vi "Autonomous Independent.vi"   [LabVIEW 2017]
doc: "This VI is called when autonomous begins, and will automatically be terminated when autonomous ends. You can carry out timed or sensor driven robot movement independently without needing to return to the caller."
uses:
  <vilib>/Rock Robotics/WPI/Solenoid/WPI_SolenoidValue.ctl
  <vilib>/Rock Robotics/Network Tables/NT Read String.vi
  <vilib>/Rock Robotics/WPI/Solenoid/WPI_SolenoidSetEnum.vi
  Robot Global Data.vi
  <vilib>/Rock Robotics/WPI/Utilities/WPI_GetSetVariantRefNum.vi
  <vilib>/Rock Robotics/WPI/ThirdParty/Phoenix-LabVIEW/Motor Controller/Get/CTRE_Phoenix_MotorController_GetQuadratureData.vi
panel:
  # "Be sure to right-click and choose Data Operations>>Make Current Value default if you want to save the array values with the VI"
types:
  T1 = typedef "WPI_SolenoidValue.ctl" = enum16{"Off", "On", "Forward", "Reverse"}
  T2 = typedef "WPI_RobotDriveDevRef.ctl" = cluster{"DevStatus":errorcluster, "Motors[]":T3[], "Square Inputs":bool, "Max Output":dbl}
  T3 = typedef "WPI_MotorControlDeviceRef.ctl" = cluster{"DeviceStatus":errorcluster, "Type":T4, "PWM":cluster{"PWM Channel":T5, "DeadBand":T6}, "CAN":cluster{"Device Number":u8, "SetOutput VI Ref":variant, "GetOutput VI Ref":variant, "Enable VI Ref":variant, "Disable VI Ref":variant, "Data":variant}, "Invert":bool, "DIO PWM":cluster{"PWM \"Enable\" Channel":T5, "DIOChannel":T7, "PWM Rate":dbl}}
  T4 = typedef "WPI_MotorControlType.ctl" = enum16{"PWM", "CAN", "DIO PWM"}
  T5 = typedef "FPGA_DIOPWMChannel.ctl" = enum8{"PWM 0", "PWM 1", "PWM 2", "PWM 3", "PWM 4", "PWM 5", "PWM 6", "PWM 7", "PWM 8", "PWM 9", "PWM MXP 0", "PWM MXP 1", "PWM MXP 2", "PWM MXP 3", "PWM MXP 4", "PWM MXP 5", "PWM MXP 6", "PWM MXP 7", "PWM MXP 8", "PWM MXP 9", "Invalid"}
  T6 = typedef "WPI_PWMDeadband.ctl" = cluster{"Name":string, "maxPositivePwm":i32, "minPositivePwm":i32, "centerPwm":i32, "maxNegativePwm":i32, "minNegativePwm":i32, "angularRange":u16}
  T7 = typedef "FPGA_DIOChannel.ctl" = enum8{"DIO 0", "DIO 1", "DIO 2", "DIO 3", "DIO 4", "DIO 5", "DIO 6", "DIO 7", "DIO 8", "DIO 9", "DIO MXP 0", "DIO MXP 1", "DIO MXP 2", "DIO MXP 3", "DIO MXP 4", "DIO MXP 5", "DIO MXP 6", "DIO MXP 7", "DIO MXP 8", "DIO MXP 9", "DIO MXP 10", "DIO MXP 11", "DIO MXP 12", "DIO MXP 13", "DIO MXP 14", "DIO MXP 15", "SPI Port CS1", "SPI Port CS2", "SPI Port CS3", "SPI Port MISO", "SPI Port MOSI", "Invalid"}
  T8 = cluster{"Yaw":dbl, "Roll":dbl, "Pitch":dbl, "Heading":dbl, "Fused Heading":dbl}
  T9 = typedef "WPI_SolenoidDevRef.ctl" = cluster{"DevStatus":errorcluster, "Pneumatics Control Module":u8, "Forward Solenoid Channel":T10, "Reverse Solenoid Channel":T10}
  T10 = typedef "WPI_SolenoidChannel.ctl" = enum8{"Solenoid 0", "Solenoid 1", "Solenoid 2", "Solenoid 3", "Solenoid 4", "Solenoid 5", "Solenoid 6", "Solenoid 7", "Invalid"}
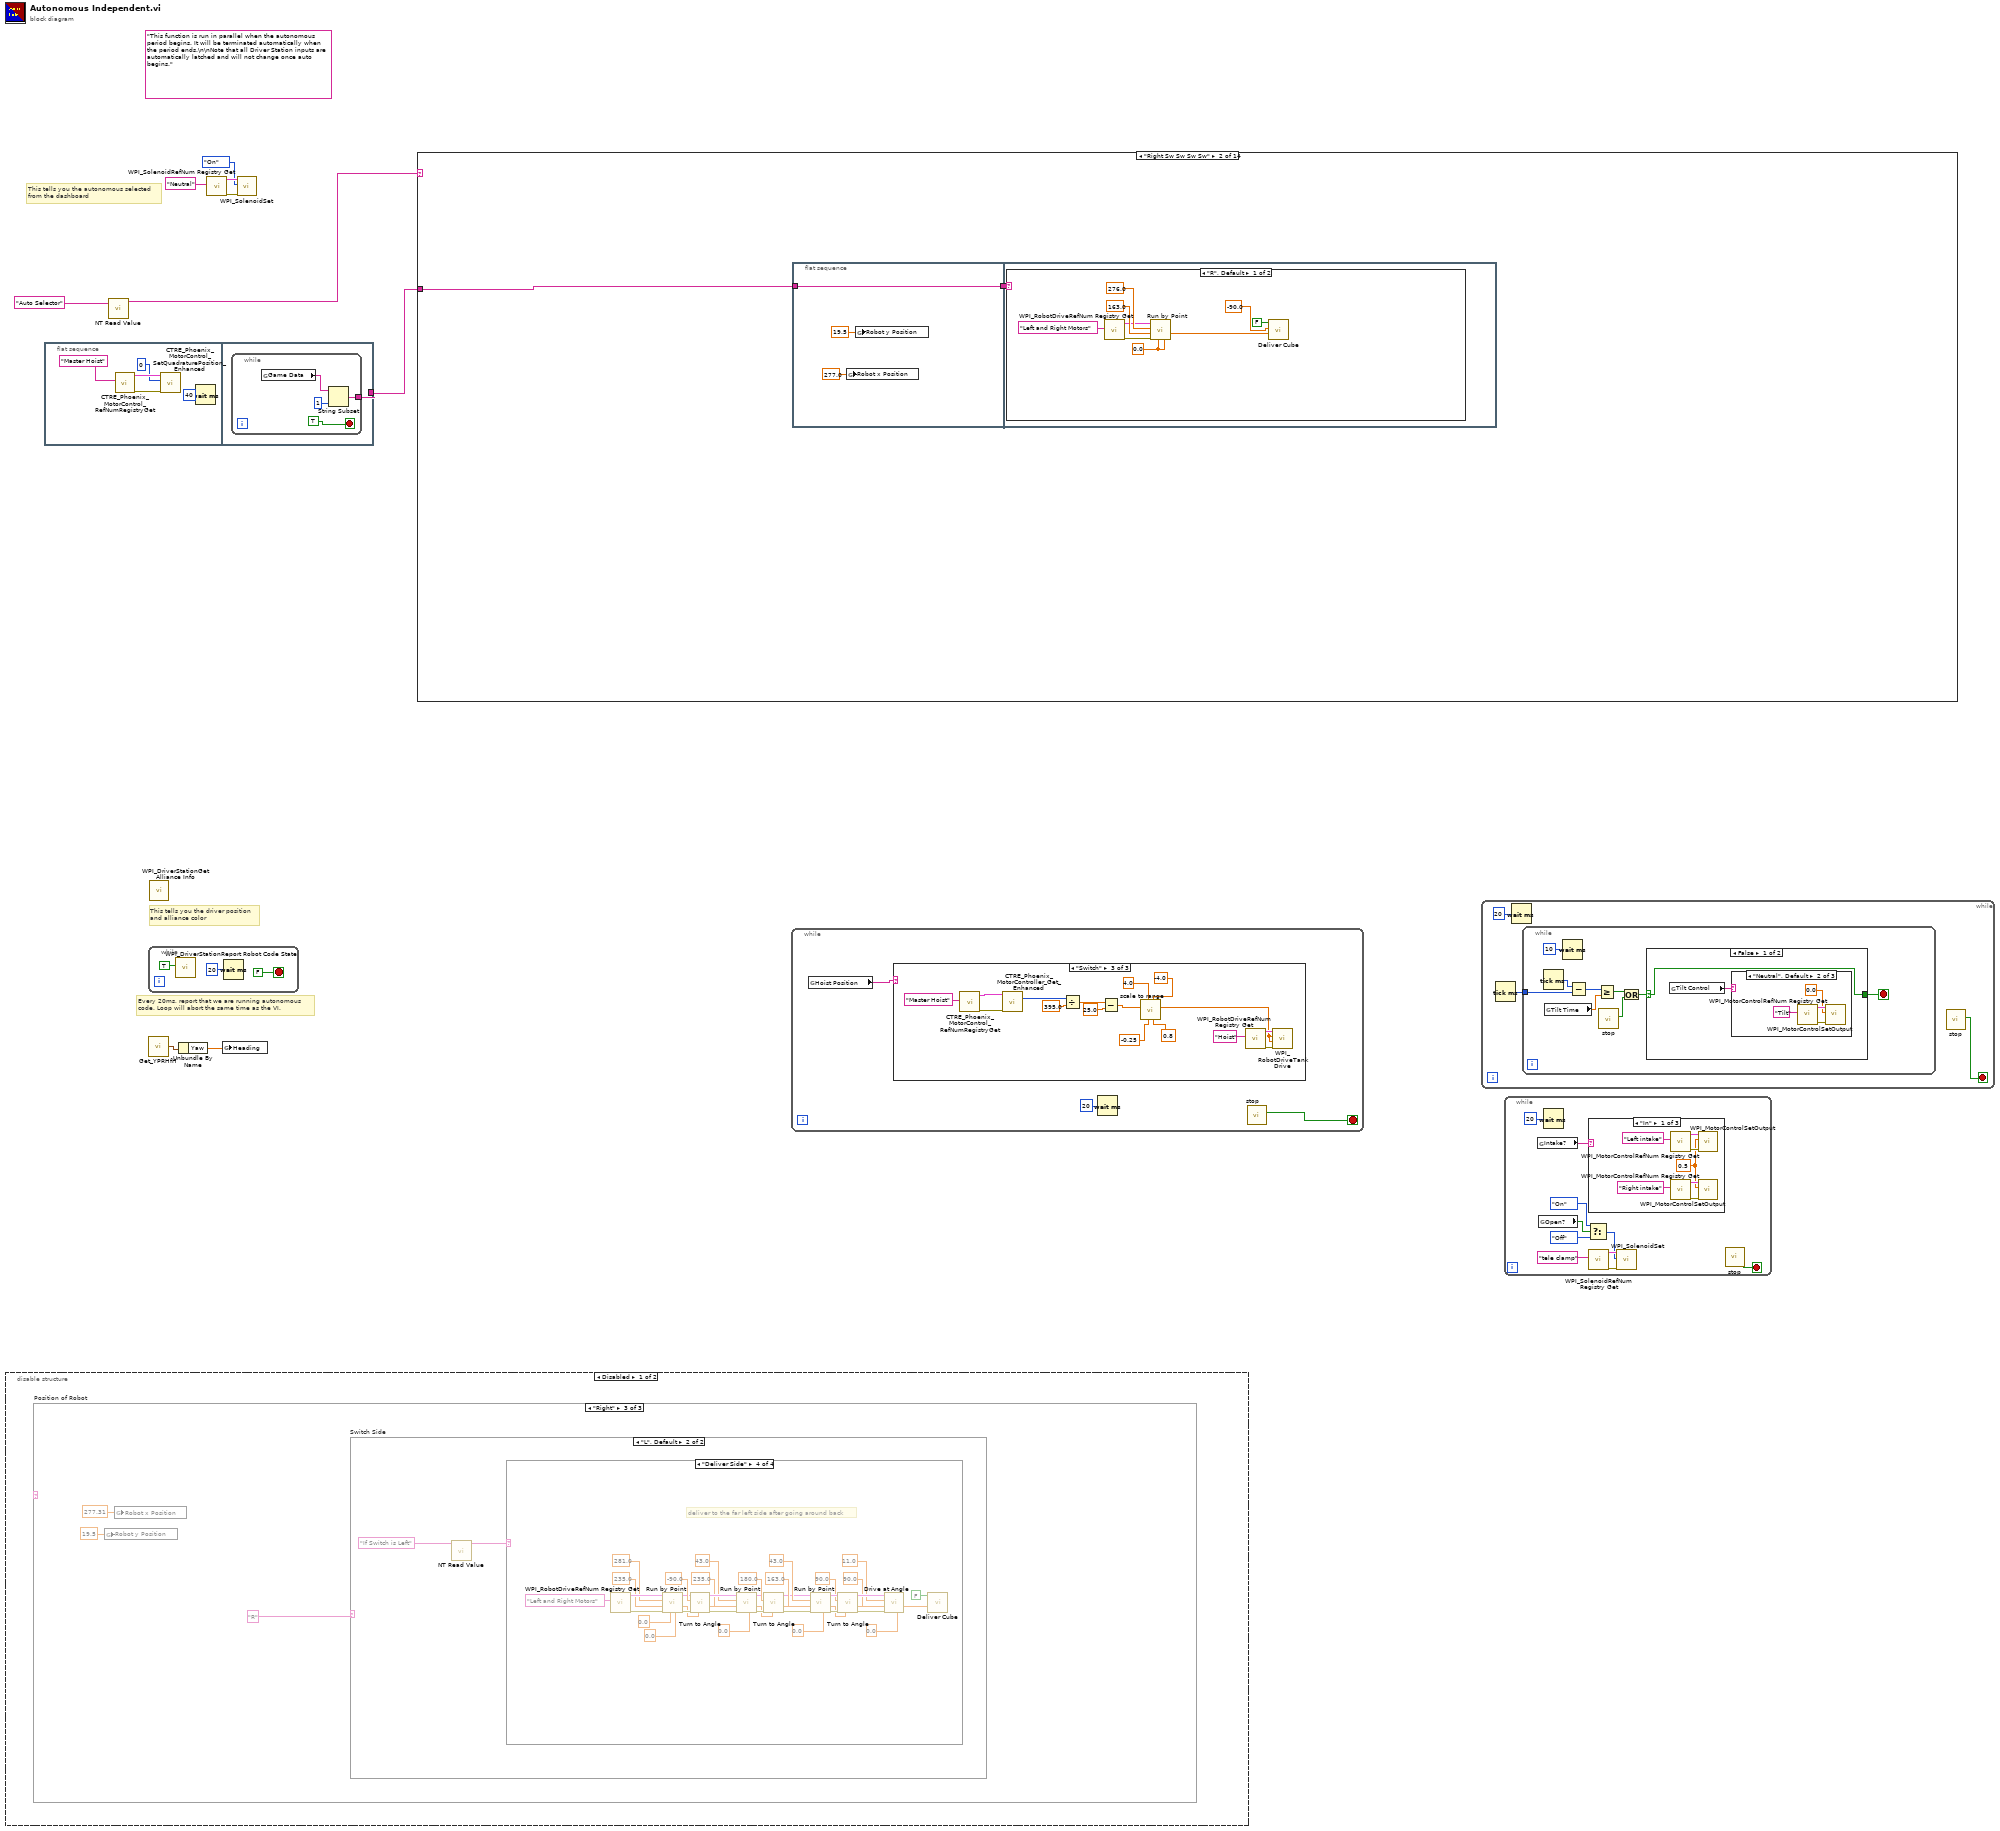
[diagram p0: block diagram]
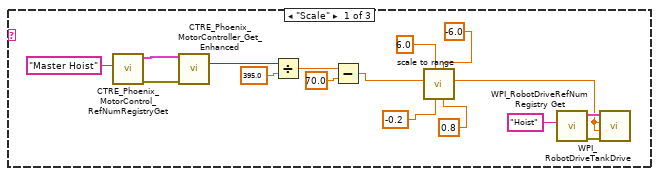
[diagram p2: hidden frame]
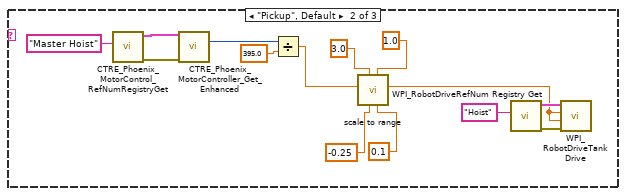
[diagram p3: hidden frame]
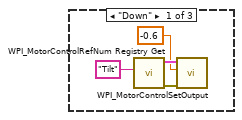
[diagram p4: hidden frame]
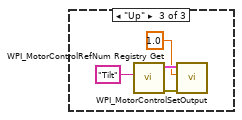
[diagram p5: hidden frame]
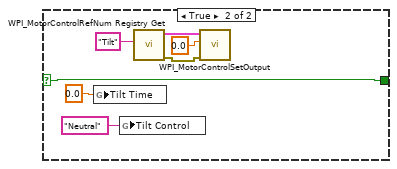
[diagram p6: hidden frame]
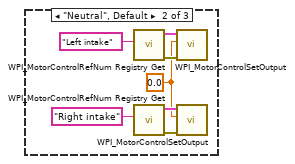
[diagram p7: hidden frame]
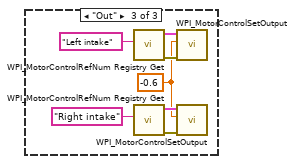
[diagram p8: hidden frame]
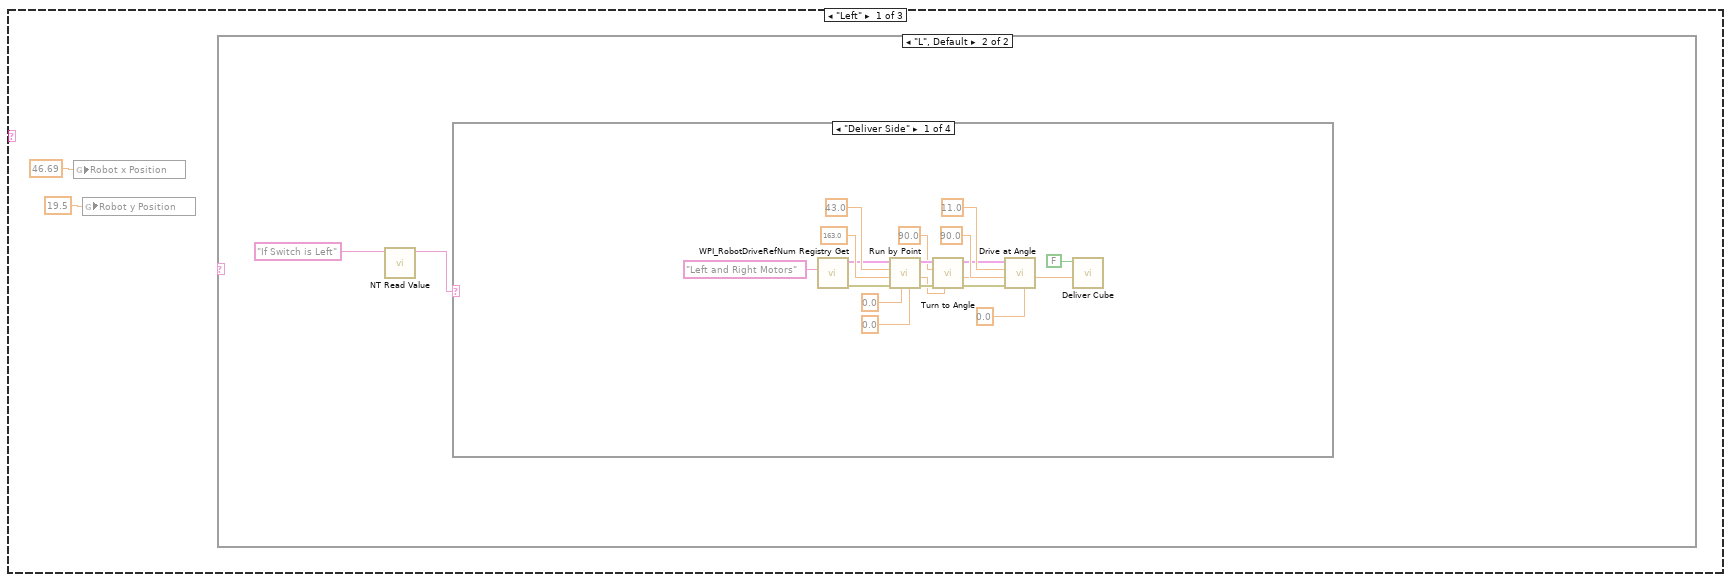
[diagram p9: hidden frame]
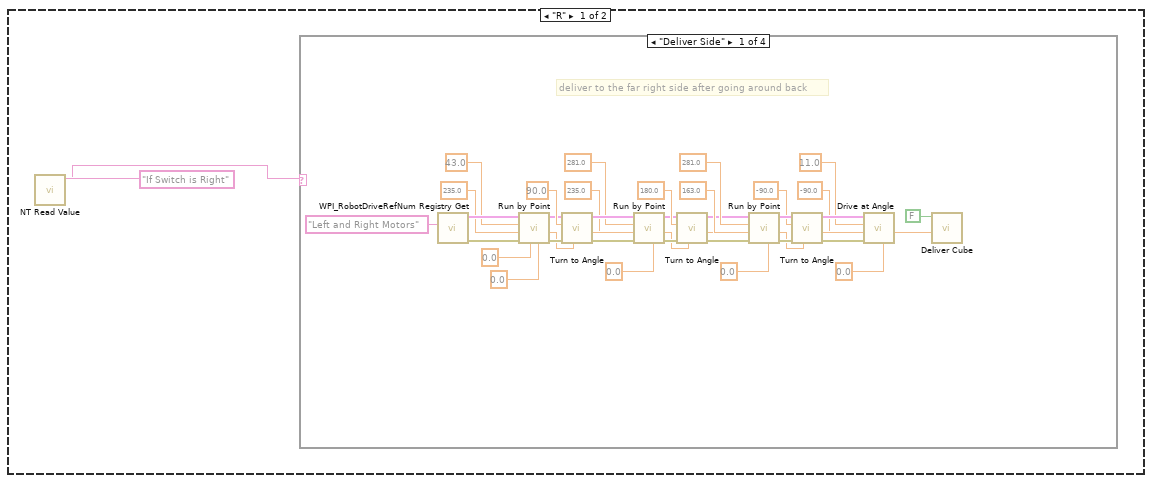
[diagram p10: hidden frame]
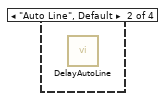
[diagram p11: hidden frame]
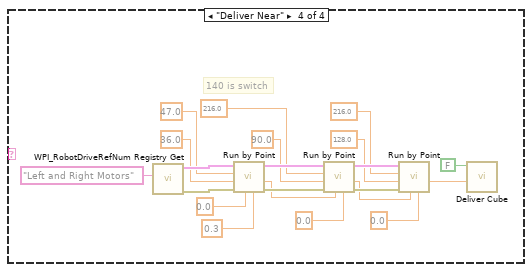
[diagram p13: hidden frame]
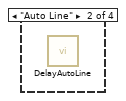
[diagram p14: hidden frame]
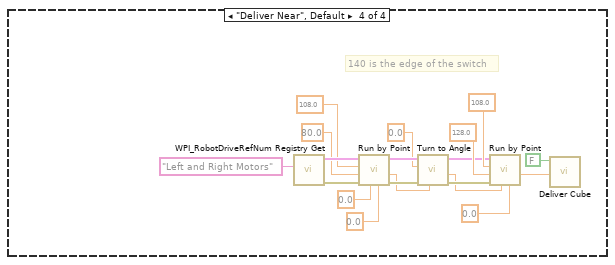
[diagram p16: hidden frame]
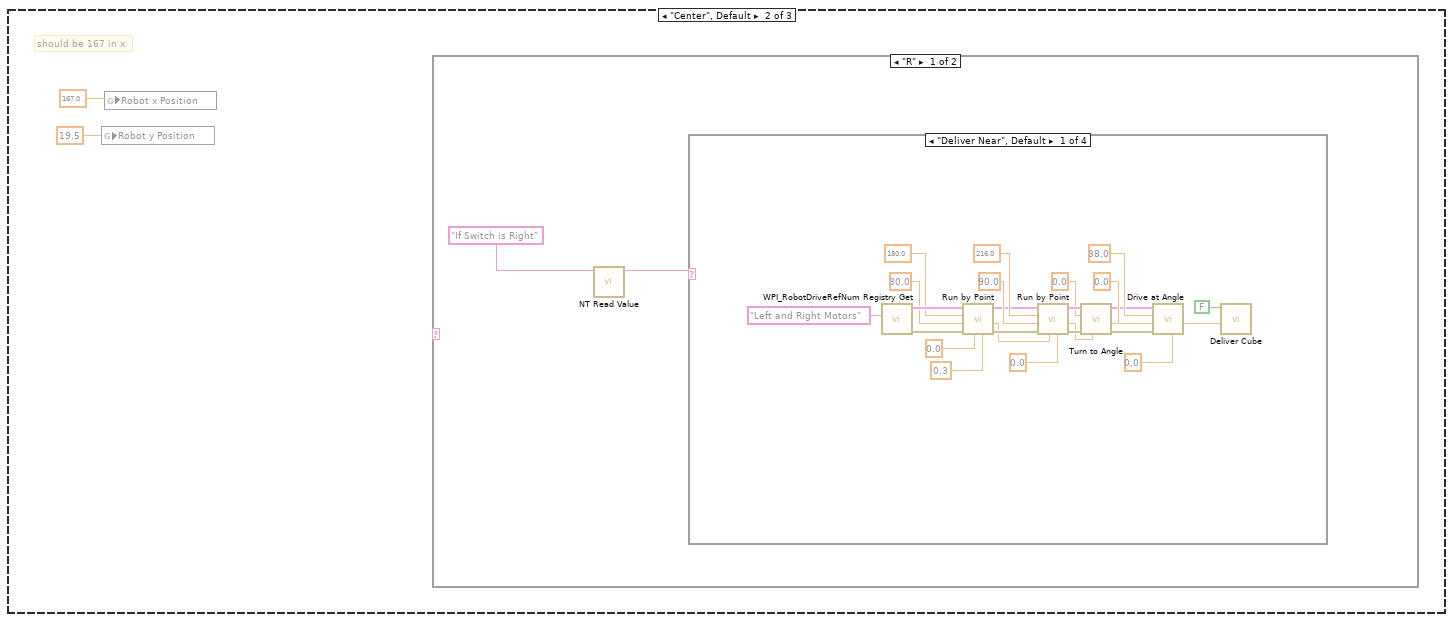
[diagram p17: hidden frame]
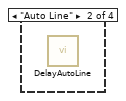
[diagram p18: hidden frame]
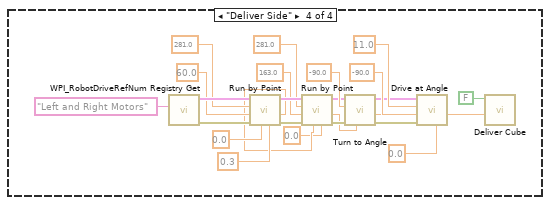
[diagram p20: hidden frame]
diagram:
  (unwired) "This function is run in parallel when the autonomous period begins. It will be terminated automatically when the period ends.\n\nNote that all Driver Station inputs are automatically latched and will not change once auto begins."
  # "This tells you the autonomous selected\nfrom the dashboard"
  # "Every 20ms, report that we are running autonomous\ncode. Loop will abort the same time as the VI."
  # "This tells you the driver position\nand alliance color"
  n1 = disable-structure shown="Disabled" {
    frame Disabled {
      n2 = case "Position of Robot" shown="\"Right\"" {
        selector: _ -> [_ _ _]
        frame "Left" {
          n3 = global write "Robot Global Data.vi" "Robot x Position"(46.69) -> ()
          n4 = global write "Robot Global Data.vi" "Robot y Position"(19.5) -> ()
          n5 = case shown="\"L\", Default" {
            selector: _ -> [_ _]
            frame "R" {
              n6 = call-poly <vilib>:"NT Read Value.vi"("Name"="If Switch is Right") -> ("String"=w12:string)  [unwired: 9 in, 1 out]
              n7 = case shown="\"Deliver Side\"" w12 {
                frame "Deliver Side" {
                  # "deliver to the far right side after going around back"
                  n8 = call <vilib>:"WPI_RobotDriveRefNum Registry Get.vi"("refnum name"="Left and Right Motors") -> ("error out"=w49:errorcluster, "RobotDriveDevRef"=w50:T2)  [unwired: 9 in]
                  n9 = call "Run by Point.vi"("end Power"=0.0 ("final power"), "Power in"=0.0 ("power in"), "error in (no error)"=w49, "y"=235.0, "x"=43.0, "RobotDriveDevRef"=w50) -> ("error out"=w40:errorcluster, "power out"=w39:dbl, "refnum"=w41:T2)  [unwired: 3 in]
                  n10 = call "Turn to Angle.vi"("in power"=w39, "error in (no error)"=w40, "Angle"=90.0 ("x"), "RobotDriveDevRef"=w41) -> ("error out"=w34:errorcluster, "out power"=w32:dbl, "ref Num"=w33:T2)  [unwired: 5 in]
                  n11 = call "Run by Point.vi"("end Power"=0.0, "Power in"=w32, "error in (no error)"=w34, "y"=235.0, "x"=281.0, "RobotDriveDevRef"=w33) -> ("error out"=w28:errorcluster, "power out"=w14:dbl, "refnum"=w29:T2)  [unwired: 3 in]
                  n12 = call "Turn to Angle.vi"("in power"=w14, "error in (no error)"=w28, "Angle"=180.0, "RobotDriveDevRef"=w29) -> ("error out"=w37:errorcluster, "out power"=w38:dbl, "ref Num"=w36:T2)  [unwired: 5 in]
                  n13 = call "Run by Point.vi"("end Power"=0.0 ("final power"), "Power in"=w38, "error in (no error)"=w37, "y"=163.0, "x"=281.0, "RobotDriveDevRef"=w36) -> ("error out"=w25:errorcluster, "power out"=w24:dbl, "refnum"=w26:T2)  [unwired: 3 in]
                  n14 = call "Turn to Angle.vi"("in power"=w24, "error in (no error)"=w25, "Angle"=-90.0, "RobotDriveDevRef"=w26) -> ("error out"=w21:errorcluster, "out power"=w20:dbl, "ref Num"=w22:T2)  [unwired: 5 in]
                  n15 = call "Drive at Angle.vi"("end power"=0.0, "Begin power"=w20, "error in (no error)"=w21, "Angle"=-90.0, "Distance"=11.0, "RobotDriveDevRef"=w22) -> ("power out"=w16:dbl)  [unwired: 3 in, 2 out]
                  n16 = call "Deliver Cube.vi"("run?"=w16, "Scale?"=FALSE) -> ()  [unwired: 9 in, 1 out]
                }
                frame "Auto Line", Default {
                  n17 = call "DelayAutoLine.vi"() -> ()  [unwired: 12 in]
                }
                frame "Scale" {
                }
                frame "Deliver Near" {
                  # "140 is switch"
                  n18 = call <vilib>:"WPI_RobotDriveRefNum Registry Get.vi"("refnum name"="Left and Right Motors") -> ("error out"=w70:errorcluster, "RobotDriveDevRef"=w71:T2)  [unwired: 9 in]
                  n19 = call "Run by Point.vi"("end Power"=0.3 ("final power"), "Power in"=0.0 ("power in"), "error in (no error)"=w70, "y"=36.0, "x"=47.0, "RobotDriveDevRef"=w71) -> ("error out"=w66:errorcluster, "power out"=w57:dbl, "refnum"=w67:T2)  [unwired: 3 in]
                  n20 = call "Run by Point.vi"("end Power"=0.0 ("final power"), "Power in"=w57, "error in (no error)"=w66, "y"=90.0, "x"=216.0, "RobotDriveDevRef"=w67) -> ("error out"=w64:errorcluster, "power out"=w63:dbl, "refnum"=w65:T2)  [unwired: 3 in]
                  n21 = call "Run by Point.vi"("end Power"=0.0 ("final power"), "Power in"=w63, "error in (no error)"=w64, "y"=128.0, "x"=216.0, "RobotDriveDevRef"=w65) -> ("power out"=w55:dbl)  [unwired: 3 in, 2 out]
                  n22 = call "Deliver Cube.vi"("run?"=w55, "Scale?"=FALSE) -> ()  [unwired: 9 in, 1 out]
                }
              }
            }
            frame "L", Default {
              n23 = call-poly <vilib>:"NT Read Value.vi"("Name"="If Switch is Left") -> ("String"=w74:string)  [unwired: 9 in, 1 out]
              n24 = case shown="\"Deliver Side\"" w74 {
                frame "Deliver Side" {
                  n25 = call <vilib>:"WPI_RobotDriveRefNum Registry Get.vi"("refnum name"="Left and Right Motors") -> ("error out"=w77:errorcluster, "RobotDriveDevRef"=w78:T2)  [unwired: 9 in]
                  n26 = call "Run by Point.vi"("end Power"=0.0 ("final power"), "Power in"=0.0, "error in (no error)"=w77, "y"=163.0 ("x"), "x"=43.0 ("y"), "RobotDriveDevRef"=w78) -> ("error out"=w87:errorcluster, "power out"=w82:dbl, "refnum"=w84:T2)  [unwired: 3 in]
                  n27 = call "Turn to Angle.vi"("in power"=w82, "error in (no error)"=w87, "Angle"=90.0, "RobotDriveDevRef"=w84) -> ("error out"=w86:errorcluster, "out power"=w81:dbl, "ref Num"=w85:T2)  [unwired: 5 in]
                  n28 = call "Drive at Angle.vi"("end power"=0.0, "Begin power"=w81, "error in (no error)"=w86, "Angle"=90.0, "Distance"=11.0, "RobotDriveDevRef"=w85) -> ("power out"=w80:dbl)  [unwired: 3 in, 2 out]
                  n29 = call "Deliver Cube.vi"("run?"=w80, "Scale?"=FALSE) -> ()  [unwired: 9 in, 1 out]
                }
                frame "Auto Line" {
                  n30 = call "DelayAutoLine.vi"() -> ()  [unwired: 12 in]
                }
                frame "Scale" {
                }
                frame "Deliver Near", Default {
                  # "140 is the edge of the switch"
                  n31 = call <vilib>:"WPI_RobotDriveRefNum Registry Get.vi"("refnum name"="Left and Right Motors") -> ("error out"=w108:errorcluster, "RobotDriveDevRef"=w109:T2)  [unwired: 9 in]
                  n32 = call "Run by Point.vi"("end Power"=0.0 ("end power"), "Power in"=0.0 ("end speed"), "error in (no error)"=w108, "y"=80.0 ("Angle"), "x"=108.0 ("Distance"), "RobotDriveDevRef"=w109) -> ("error out"=w100:errorcluster, "power out"=w99:dbl, "refnum"=w103:T2)  [unwired: 3 in]
                  n33 = call "Turn to Angle.vi"("in power"=w99, "error in (no error)"=w100, "Angle"=0.0 ("y"), "RobotDriveDevRef"=w103) -> ("error out"=w101:errorcluster, "out power"=w97:dbl, "ref Num"=w102:T2)  [unwired: 5 in]
                  n34 = call "Run by Point.vi"("end Power"=0.0, "Power in"=w97, "error in (no error)"=w101, "y"=128.0, "x"=108.0, "RobotDriveDevRef"=w102) -> ("power out"=w96:dbl)  [unwired: 3 in, 2 out]
                  n35 = call "Deliver Cube.vi"("run?"=w96, "Scale?"=FALSE) -> ()  [unwired: 9 in, 1 out]
                }
              }
            }
          }
        }
        frame "Center", Default {
          # "should be 167 in x"
          n36 = global write "Robot Global Data.vi" "Robot y Position"(19.5) -> ()
          n37 = global write "Robot Global Data.vi" "Robot x Position"(167.0) -> ()
          n38 = case shown="\"R\"" {
            selector: _ -> [_ _]
            frame "R" {
              n39 = call-poly <vilib>:"NT Read Value.vi"("Name"="If Switch is Right") -> ("String"=w116:string)  [unwired: 9 in, 1 out]
              n40 = case shown="\"Deliver Near\", Default" w116 {
                frame "Deliver Near", Default {
                  n41 = call <vilib>:"WPI_RobotDriveRefNum Registry Get.vi"("refnum name"="Left and Right Motors") -> ("error out"=w133:errorcluster, "RobotDriveDevRef"=w134:T2)  [unwired: 9 in]
                  n42 = call "Run by Point.vi"("end Power"=0.3 ("Power in"), "Power in"=0.0, "error in (no error)"=w133, "y"=30.0, "x"=180.0, "RobotDriveDevRef"=w134) -> ("error out"=w132:errorcluster, "power out"=w130:dbl, "refnum"=w131:T2)  [unwired: 3 in]
                  n43 = call "Run by Point.vi"("end Power"=0.0, "Power in"=w130, "error in (no error)"=w132, "y"=90.0, "x"=216.0, "RobotDriveDevRef"=w131) -> ("error out"=w125:errorcluster, "power out"=w123:dbl, "refnum"=w124:T2)  [unwired: 3 in]
                  n44 = call "Turn to Angle.vi"("in power"=w123, "error in (no error)"=w125, "Angle"=0.0, "RobotDriveDevRef"=w124) -> ("error out"=w121:errorcluster, "out power"=w119:dbl, "ref Num"=w120:T2)  [unwired: 5 in]
                  n45 = call "Drive at Angle.vi"("end power"=0.0 ("final power"), "Begin power"=w119, "error in (no error)"=w121, "Angle"=0.0 ("x"), "Distance"=38.0 ("y"), "RobotDriveDevRef"=w120) -> ("power out"=w118:dbl)  [unwired: 3 in, 2 out]
                  n46 = call "Deliver Cube.vi"("run?"=w118, "Scale?"=FALSE) -> ()  [unwired: 9 in, 1 out]
                }
                frame "Auto Line" {
                  n47 = call "DelayAutoLine.vi"() -> ()  [unwired: 12 in]
                }
                frame "Scale" {
                }
                frame "Deliver Side" {
                  n48 = call <vilib>:"WPI_RobotDriveRefNum Registry Get.vi"("refnum name"="Left and Right Motors") -> ("error out"=w156:errorcluster, "RobotDriveDevRef"=w166:T2)  [unwired: 9 in]
                  n49 = call "Run by Point.vi"("end Power"=0.3 ("final power"), "Power in"=0.0 ("power in"), "error in (no error)"=w156, "y"=60.0, "x"=281.0, "RobotDriveDevRef"=w166) -> ("error out"=w151:errorcluster, "power out"=w150:dbl, "refnum"=w152:T2)  [unwired: 3 in]
                  n50 = call "Run by Point.vi"("end Power"=0.0, "Power in"=w150, "error in (no error)"=w151, "y"=163.0, "x"=281.0, "RobotDriveDevRef"=w152) -> ("error out"=w146:errorcluster, "power out"=w145:dbl, "refnum"=w147:T2)  [unwired: 3 in]
                  n51 = call "Turn to Angle.vi"("in power"=w145, "error in (no error)"=w146, "Angle"=-90.0 ("x"), "RobotDriveDevRef"=w147) -> ("error out"=w153:errorcluster, "out power"=w144:dbl, "ref Num"=w154:T2)  [unwired: 5 in]
                  n52 = call "Drive at Angle.vi"("end power"=0.0, "Begin power"=w144, "error in (no error)"=w153, "Angle"=-90.0, "Distance"=11.0, "RobotDriveDevRef"=w154) -> ("power out"=w158:dbl)  [unwired: 3 in, 2 out]
                  n53 = call "Deliver Cube.vi"("run?"=w158, "Scale?"=FALSE) -> ()  [unwired: 9 in, 1 out]
                }
              }
            }
            frame "L", Default {
              n54 = call-poly <vilib>:"NT Read Value.vi"("Name"="If Switch is Left") -> ("String"=w168:string)  [unwired: 9 in, 1 out]
              n55 = case shown="\"Deliver Near\", Default" w168 {
                frame "Deliver Near", Default {
                  n56 = call <vilib>:"WPI_RobotDriveRefNum Registry Get.vi"("refnum name"="Left and Right Motors") -> ("error out"=w185:errorcluster, "RobotDriveDevRef"=w186:T2)  [unwired: 9 in]
                  n57 = call "Run by Point.vi"("end Power"=0.3 ("Power in"), "Power in"=0.0, "error in (no error)"=w185, "y"=30.0, "x"=150.0, "RobotDriveDevRef"=w186) -> ("error out"=w184:errorcluster, "power out"=w182:dbl, "refnum"=w183:T2)  [unwired: 3 in]
                  n58 = call "Run by Point.vi"("end Power"=0.0, "Power in"=w182, "error in (no error)"=w184, "y"=90.0, "x"=108.0, "RobotDriveDevRef"=w183) -> ("error out"=w177:errorcluster, "power out"=w175:dbl, "refnum"=w176:T2)  [unwired: 3 in]
                  n59 = call "Turn to Angle.vi"("in power"=w175, "error in (no error)"=w177, "Angle"=0.0, "RobotDriveDevRef"=w176) -> ("error out"=w173:errorcluster, "out power"=w171:dbl, "ref Num"=w172:T2)  [unwired: 5 in]
                  n60 = call "Drive at Angle.vi"("end power"=0.0 ("final power"), "Begin power"=w171, "error in (no error)"=w173, "Angle"=0.0 ("x"), "Distance"=38.0 ("y"), "RobotDriveDevRef"=w172) -> ("power out"=w170:dbl)  [unwired: 3 in, 2 out]
                  n61 = call "Deliver Cube.vi"("run?"=w170, "Scale?"=FALSE) -> ()  [unwired: 9 in, 1 out]
                }
                frame "Auto Line" {
                  n62 = call "DelayAutoLine.vi"() -> ()  [unwired: 12 in]
                }
                frame "Scale" {
                }
                frame "Deliver Side" {
                  n63 = call <vilib>:"WPI_RobotDriveRefNum Registry Get.vi"("refnum name"="Left and Right Motors") -> ("error out"=w208:errorcluster, "RobotDriveDevRef"=w218:T2)  [unwired: 9 in]
                  n64 = call "Run by Point.vi"("end Power"=0.3 ("final power"), "Power in"=0.0 ("power in"), "error in (no error)"=w208, "y"=60.0, "x"=43.0, "RobotDriveDevRef"=w218) -> ("error out"=w203:errorcluster, "power out"=w202:dbl, "refnum"=w204:T2)  [unwired: 3 in]
                  n65 = call "Run by Point.vi"("end Power"=0.0, "Power in"=w202, "error in (no error)"=w203, "y"=163.0, "x"=43.0, "RobotDriveDevRef"=w204) -> ("error out"=w198:errorcluster, "power out"=w197:dbl, "refnum"=w199:T2)  [unwired: 3 in]
                  n66 = call "Turn to Angle.vi"("in power"=w197, "error in (no error)"=w198, "Angle"=90.0 ("x"), "RobotDriveDevRef"=w199) -> ("error out"=w205:errorcluster, "out power"=w196:dbl, "ref Num"=w206:T2)  [unwired: 5 in]
                  n67 = call "Drive at Angle.vi"("end power"=0.0, "Begin power"=w196, "error in (no error)"=w205, "Angle"=90.0, "Distance"=11.0, "RobotDriveDevRef"=w206) -> ("power out"=w210:dbl)  [unwired: 3 in, 2 out]
                  n68 = call "Deliver Cube.vi"("run?"=w210, "Scale?"=FALSE) -> ()  [unwired: 9 in, 1 out]
                }
              }
            }
          }
        }
        frame "Right" {
          n69 = global write "Robot Global Data.vi" "Robot y Position"(19.5) -> ()
          n70 = global write "Robot Global Data.vi" "Robot x Position"(277.31) -> ()
          n71 = case "Switch Side" shown="\"L\", Default" "R" {
            frame "R" {
              n72 = call-poly <vilib>:"NT Read Value.vi"("Name"="If Switch is Right") -> ()  [unwired: 9 in, 2 out]
              n73 = case "What Program to Run" shown="\"Deliver Side\"" "Auto Line" {
                frame "Deliver Near", Default {
                  n74 = call <vilib>:"WPI_RobotDriveRefNum Registry Get.vi"("refnum name"="Left and Right Motors") -> ("error out"=w240:errorcluster, "RobotDriveDevRef"=w241:T2)  [unwired: 9 in]
                  n75 = call "Run by Point.vi"("end Power"=0.3 ("Power in"), "Power in"=0.0, "error in (no error)"=w240, "y"=30.0, "x"=250.0, "RobotDriveDevRef"=w241) -> ("error out"=w239:errorcluster, "power out"=w237:dbl, "refnum"=w238:T2)  [unwired: 3 in]
                  n76 = call "Run by Point.vi"("end Power"=0.0, "Power in"=w237, "error in (no error)"=w239, "y"=90.0, "x"=216.0, "RobotDriveDevRef"=w238) -> ("error out"=w232:errorcluster, "power out"=w230:dbl, "refnum"=w231:T2)  [unwired: 3 in]
                  n77 = call "Turn to Angle.vi"("in power"=w230, "error in (no error)"=w232, "Angle"=0.0, "RobotDriveDevRef"=w231) -> ("error out"=w228:errorcluster, "out power"=w226:dbl, "ref Num"=w227:T2)  [unwired: 5 in]
                  n78 = call "Drive at Angle.vi"("end power"=0.0 ("final power"), "Begin power"=w226, "error in (no error)"=w228, "Angle"=0.0 ("x"), "Distance"=38.0 ("y"), "RobotDriveDevRef"=w227) -> ("power out"=w225:dbl)  [unwired: 3 in, 2 out]
                  n79 = call "Deliver Cube.vi"("run?"=w225, "Scale?"=FALSE) -> ()  [unwired: 9 in, 1 out]
                }
                frame "Auto Line" {
                  n80 = call "DelayAutoLine.vi"() -> ()  [unwired: 12 in]
                }
                frame "Scale" {
                }
                frame "Deliver Side" {
                  n81 = call <vilib>:"WPI_RobotDriveRefNum Registry Get.vi"("refnum name"="Left and Right Motors") -> ("error out"=w250:errorcluster, "RobotDriveDevRef"=w251:T2)  [unwired: 9 in]
                  n82 = call "Run by Point.vi"("end Power"=0.0, "error in (no error)"=w250, "y"=163.0, "x"=281.0, "RobotDriveDevRef"=w251) -> ("error out"=w255:errorcluster, "power out"=w254:dbl, "refnum"=w256:T2)  [unwired: 4 in]
                  n83 = call "Turn to Angle.vi"("in power"=w254, "error in (no error)"=w255, "Angle"=-90.0 ("x"), "RobotDriveDevRef"=w256) -> ("error out"=w259:errorcluster, "out power"=w253:dbl, "ref Num"=w260:T2)  [unwired: 5 in]
                  n84 = call "Drive at Angle.vi"("end power"=0.0, "Begin power"=w253, "error in (no error)"=w259, "Angle"=-90.0, "Distance"=11.0, "RobotDriveDevRef"=w260) -> ("power out"=w263:dbl)  [unwired: 3 in, 2 out]
                  n85 = call "Deliver Cube.vi"("run?"=w263, "Scale?"=FALSE) -> ()  [unwired: 9 in, 1 out]
                }
              }
            }
            frame "L", Default {
              n86 = call-poly <vilib>:"NT Read Value.vi"("Name"="If Switch is Left") -> ("String"=w268:string)  [unwired: 9 in, 1 out]
              n87 = case shown="\"Deliver Side\"" w268 {
                frame "Deliver Near" {
                  # "140 is switch"
                  n88 = call <vilib>:"WPI_RobotDriveRefNum Registry Get.vi"("refnum name"="Left and Right Motors") -> ("error out"=w287:errorcluster, "RobotDriveDevRef"=w288:T2)  [unwired: 9 in]
                  n89 = call "Run by Point.vi"("end Power"=0.3 ("final power"), "Power in"=0.0 ("power in"), "error in (no error)"=w287, "y"=45.0, "x"=108.0, "RobotDriveDevRef"=w288) -> ("error out"=w283:errorcluster, "power out"=w274:dbl, "refnum"=w284:T2)  [unwired: 3 in]
                  n90 = call "Run by Point.vi"("end Power"=0.3 ("final power"), "Power in"=w274, "error in (no error)"=w283, "y"=90.0, "x"=108.0, "RobotDriveDevRef"=w284) -> ("error out"=w281:errorcluster, "power out"=w280:dbl, "refnum"=w282:T2)  [unwired: 3 in]
                  n91 = call "Drive at Angle.vi"("end power"=0.0 ("final power"), "Begin power"=w280, "error in (no error)"=w281, "Angle"=0.0 ("y"), "Distance"=38.0 ("x"), "RobotDriveDevRef"=w282) -> ("power out"=w272:dbl)  [unwired: 3 in, 2 out]
                  n92 = call "Deliver Cube.vi"("run?"=w272, "Scale?"=FALSE) -> ()  [unwired: 9 in, 1 out]
                }
                frame "Auto Line", Default {
                  n93 = call "DelayAutoLine.vi"() -> ()  [unwired: 12 in]
                }
                frame "Scale" {
                }
                frame "Deliver Side" {
                  # "deliver to the far left side after going around back"
                  n94 = call <vilib>:"WPI_RobotDriveRefNum Registry Get.vi"("refnum name"="Left and Right Motors") -> ("error out"=w326:errorcluster, "RobotDriveDevRef"=w327:T2)  [unwired: 9 in]
                  n95 = call "Run by Point.vi"("end Power"=0.0 ("final power"), "Power in"=0.0 ("power in"), "error in (no error)"=w326, "y"=235.0, "x"=281.0, "RobotDriveDevRef"=w327) -> ("error out"=w317:errorcluster, "power out"=w316:dbl, "refnum"=w318:T2)  [unwired: 3 in]
                  n96 = call "Turn to Angle.vi"("in power"=w316, "error in (no error)"=w317, "Angle"=-90.0 ("x"), "RobotDriveDevRef"=w318) -> ("error out"=w311:errorcluster, "out power"=w309:dbl, "ref Num"=w310:T2)  [unwired: 5 in]
                  n97 = call "Run by Point.vi"("end Power"=0.0, "Power in"=w309, "error in (no error)"=w311, "y"=235.0, "x"=43.0, "RobotDriveDevRef"=w310) -> ("error out"=w305:errorcluster, "power out"=w291:dbl, "refnum"=w306:T2)  [unwired: 3 in]
                  n98 = call "Turn to Angle.vi"("in power"=w291, "error in (no error)"=w305, "Angle"=180.0, "RobotDriveDevRef"=w306) -> ("error out"=w314:errorcluster, "out power"=w315:dbl, "ref Num"=w313:T2)  [unwired: 5 in]
                  n99 = call "Run by Point.vi"("end Power"=0.0 ("final power"), "Power in"=w315, "error in (no error)"=w314, "y"=163.0, "x"=43.0, "RobotDriveDevRef"=w313) -> ("error out"=w302:errorcluster, "power out"=w301:dbl, "refnum"=w303:T2)  [unwired: 3 in]
                  n100 = call "Turn to Angle.vi"("in power"=w301, "error in (no error)"=w302, "Angle"=90.0, "RobotDriveDevRef"=w303) -> ("error out"=w298:errorcluster, "out power"=w297:dbl, "ref Num"=w299:T2)  [unwired: 5 in]
                  n101 = call "Drive at Angle.vi"("end power"=0.0, "Begin power"=w297, "error in (no error)"=w298, "Angle"=90.0, "Distance"=11.0, "RobotDriveDevRef"=w299) -> ("power out"=w293:dbl)  [unwired: 3 in, 2 out]
                  n102 = call "Deliver Cube.vi"("run?"=w293, "Scale?"=FALSE) -> ()  [unwired: 9 in, 1 out]
                }
              }
            }
          }
        }
      }
    }
    frame Enabled {
    }
  }
  n103 = flat-sequence {
    tunnel: [w335] -> w1
    frame #0 {
      n104 = call <vilib>:"CTRE_Phoenix_MotorControl_RefNumRegistryGet.vi"("refnum name"="Master Hoist") -> ("error out"=w333:errorcluster, "PhoenixMotorControlDevRef"=w332:T3)  [unwired: 9 in]
      n105 = call <vilib>:"CTRE_Phoenix_MotorControl_SetQuadraturePosition_Enhanced.vi"("error in (no error)"=w333, "New Position"=0, "PhoenixMotorControlDevRef"=w332) -> ()  [unwired: 7 in, 2 out]
      n106 = Wait (ms)(milliseconds to wait=u32 40) -> ()  [unwired: 1 out]
    }
    frame #1 {
      n107 = while {
        tunnel: [w338] -> w335
        stop <- TRUE stop-if-true
        n108 = global read "Robot Global Data.vi" "Game Data"() -> (w337:string)
        n109 = String Subset(string=w337, length (rest)=1 ("length (rest)")) -> (substring=w338:string)  [unwired: 1 in]
      }
    }
  }
  n110 = call-poly <vilib>:"NT Read Value.vi"("Name"="Auto Selector") -> ("String"=w2:string)  [unwired: 9 in, 1 out]
  n111 = while {
    stop <- FALSE stop-if-true
    n112 = call <vilib>:"WPI_DriverStationReport Robot Code State.vi"("Autonomous"=TRUE) -> ()  [unwired: 10 in, 1 out]
    n113 = Wait (ms)(milliseconds to wait=u32 20) -> ()  [unwired: 1 out]
  }
  n114 = call <vilib>:"Get_YPRHfH.vi"() -> ("YRPHfH"=w7:T8)  [unwired: 11 in]
  n115 = call <vilib>:"WPI_DriverStationGet Alliance Info.vi"() -> ()  [unwired: 12 out]
  n116 = Unbundle By Name(w7) -> ("Yaw"=w8:dbl)
  n117 = call <vilib>:"WPI_SolenoidRefNum Registry Get.vi"("refnum name"="Neutral") -> ("error out"=w6:errorcluster, "SolenoidDevRef"=w5:T9)  [unwired: 9 in]
  n118 = global write "Robot Global Data.vi" "Heading"(w8) -> ()
  n119 = call-poly <vilib>:"WPI_SolenoidSet.vi"("error in (no error)"=w6, "Value"=WPI_SolenoidValue."On", "SolenoidDevRef"=w5) -> ()  [unwired: 7 in, 2 out]
  n120 = case shown="\"Right Sw Sw Sw Sw\"" w2 {
    tunnel: w1 -> [w344 w370 _ w417 w432 w446 w451 _ _ w579 w644 w707 w770 w833]
    frame "Center" {
      n121 = flat-sequence {
        tunnel: w344 -> [w347]
        tunnel: [w347] -> w343
        tunnel: w343 -> [w348]
        frame #0 {
          n122 = global write "Robot Global Data.vi" "Robot y Position"(19.5) -> ()
          n123 = global write "Robot Global Data.vi" "Robot x Position"(167.0) -> ()
        }
        frame #1 {
          n124 = case shown="\"L\", Default" w348 {
            frame "R" {
              n125 = call <vilib>:"WPI_RobotDriveRefNum Registry Get.vi"("refnum name"="Left and Right Motors") -> ("error out"=w354:errorcluster, "RobotDriveDevRef"=w355:T2)  [unwired: 9 in]
              n126 = call "Run by Point.vi"("end Power"=0.0, "Power in"=0.0, "error in (no error)"=w354, "y"=103.0, "x"=216.0, "RobotDriveDevRef"=w355) -> ("power out"=w353:dbl)  [unwired: 3 in, 2 out]
              n127 = call "Deliver Cube.vi"("run?"=w353, "Angle"=0.0, "Scale?"=FALSE) -> ()  [unwired: 8 in, 1 out]
            }
            frame "L", Default {
              n128 = call <vilib>:"WPI_RobotDriveRefNum Registry Get.vi"("refnum name"="Left and Right Motors") -> ("error out"=w364:errorcluster, "RobotDriveDevRef"=w365:T2)  [unwired: 9 in]
              n129 = call "Run by Point.vi"("end Power"=0.0, "Power in"=0.0, "error in (no error)"=w364, "y"=103.0, "x"=108.0, "RobotDriveDevRef"=w365) -> ("power out"=w359:dbl)  [unwired: 3 in, 2 out]
              n130 = call "Deliver Cube.vi"("run?"=w359, "Angle"=0.0, "Scale?"=FALSE) -> ()  [unwired: 8 in, 1 out]
            }
          }
        }
      }
    }
    frame "Right Sw Sw Sw Sw" {
      n131 = flat-sequence {
        tunnel: w370 -> [w373]
        tunnel: [w373] -> w369
        tunnel: w369 -> [w374]
        frame #0 {
          n132 = global write "Robot Global Data.vi" "Robot x Position"(277.0) -> ()
          n133 = global write "Robot Global Data.vi" "Robot y Position"(19.5) -> ()
        }
        frame #1 {
          n134 = case shown="\"R\", Default" w374 {
            frame "R", Default {
              w376 = 0.0 ("end Power")
              n135 = call <vilib>:"WPI_RobotDriveRefNum Registry Get.vi"("refnum name"="Left and Right Motors") -> ("error out"=w378:errorcluster, "RobotDriveDevRef"=w379:T2)  [unwired: 9 in]
              n136 = call "Run by Point.vi"("end Power"=w376, "Power in"=w376, "error in (no error)"=w378, "y"=163.0, "x"=276.0, "RobotDriveDevRef"=w379) -> ("power out"=w377:dbl)  [unwired: 3 in, 2 out]
              n137 = call "Deliver Cube.vi"("run?"=w377, "Angle"=-90.0 ("x"), "Scale?"=FALSE) -> ()  [unwired: 8 in, 1 out]
            }
            frame "L" {
              # "deliver to the far left side after going around back"
              n138 = call <vilib>:"WPI_RobotDriveRefNum Registry Get.vi"("refnum name"="Left and Right Motors") -> ("error out"=w410:errorcluster, "RobotDriveDevRef"=w411:T2)  [unwired: 9 in]
              n139 = call "Run by Point.vi"("end Power"=0.0 ("final power"), "Power in"=0.0 ("power in"), "error in (no error)"=w410, "y"=235.0, "x"=281.0, "RobotDriveDevRef"=w411) -> ("error out"=w401:errorcluster, "power out"=w400:dbl, "refnum"=w402:T2)  [unwired: 3 in]
              n140 = call "Turn to Angle.vi"("in power"=w400, "error in (no error)"=w401, "Angle"=-90.0 ("x"), "RobotDriveDevRef"=w402) -> ("error out"=w395:errorcluster, "out power"=w393:dbl, "ref Num"=w394:T2)  [unwired: 5 in]
              n141 = call "Run by Point.vi"("end Power"=0.0, "Power in"=w393, "error in (no error)"=w395, "y"=235.0, "x"=43.0, "RobotDriveDevRef"=w394) -> ("error out"=w389:errorcluster, "power out"=w386:dbl, "refnum"=w390:T2)  [unwired: 3 in]
              n142 = call "Turn to Angle.vi"("in power"=w386, "error in (no error)"=w389, "Angle"=180.0, "RobotDriveDevRef"=w390) -> ("error out"=w398:errorcluster, "out power"=w399:dbl, "ref Num"=w397:T2)  [unwired: 5 in]
              n143 = call "Run by Point.vi"("end Power"=0.0 ("final power"), "Power in"=w399, "error in (no error)"=w398, "y"=163.0, "x"=48.0, "RobotDriveDevRef"=w397) -> ("power out"=w384:dbl)  [unwired: 3 in, 2 out]
              n144 = call "Deliver Cube.vi"("run?"=w384, "Angle"=90.0, "Scale?"=FALSE) -> ()  [unwired: 8 in, 1 out]
            }
          }
        }
      }
    }
    frame "Left Ln Ln Ln Ln", Default {
      n145 = flat-sequence {
        frame #0 {
          n146 = global write "Robot Global Data.vi" "Robot x Position"(46.0) -> ()
          n147 = global write "Robot Global Data.vi" "Robot y Position"(19.5) -> ()
        }
        frame #1 {
          n148 = call "DelayAutoLine.vi"() -> ()  [unwired: 12 in]
        }
      }
    }
    frame "Left Sw Sw Ln Ln" {
      n149 = flat-sequence {
        tunnel: w417 -> [w420]
        tunnel: [w420] -> w416
        tunnel: w416 -> [w421]
        frame #0 {
          n150 = global write "Robot Global Data.vi" "Robot y Position"(19.5) -> ()
          n151 = global write "Robot Global Data.vi" "Robot x Position"(46.0) -> ()
        }
        frame #1 {
          n152 = case shown="\"L\", Default" w421 {
            frame "R" {
              n153 = call "DelayAutoLine.vi"() -> ()  [unwired: 12 in]
            }
            frame "L", Default {
              n154 = call <vilib>:"WPI_RobotDriveRefNum Registry Get.vi"("refnum name"="Left and Right Motors") -> ("error out"=w425:errorcluster, "RobotDriveDevRef"=w426:T2)  [unwired: 9 in]
              n155 = call "Run by Point.vi"("end Power"=0.0 ("final power"), "Power in"=0.0, "error in (no error)"=w425, "y"=163.0 ("x"), "x"=48.0 ("y"), "RobotDriveDevRef"=w426) -> ("power out"=w422:dbl)  [unwired: 3 in, 2 out]
              n156 = call "Deliver Cube.vi"("run?"=w422, "Angle"=90.0, "Scale?"=FALSE) -> ()  [unwired: 8 in, 1 out]
            }
          }
        }
      }
    }
    frame "Right Ln Ln Sw Sw" {
      n157 = flat-sequence {
        tunnel: w432 -> [w435]
        frame #0 {
          n158 = global write "Robot Global Data.vi" "Robot y Position"(19.5) -> ()
          n159 = global write "Robot Global Data.vi" "Robot x Position"(277.0) -> ()
        }
        frame #1 {
          n160 = case shown="\"R\", Default" w435 {
            frame "R", Default {
              n161 = call <vilib>:"WPI_RobotDriveRefNum Registry Get.vi"("refnum name"="Left and Right Motors") -> ("error out"=w438:errorcluster, "RobotDriveDevRef"=w439:T2)  [unwired: 9 in]
              n162 = call "Run by Point.vi"("end Power"=0.0, "error in (no error)"=w438, "y"=163.0, "x"=276.0, "RobotDriveDevRef"=w439) -> ("power out"=w436:dbl)  [unwired: 4 in, 2 out]
              n163 = call "Deliver Cube.vi"("run?"=w436, "Angle"=-90.0 ("x"), "Scale?"=FALSE) -> ()  [unwired: 8 in, 1 out]
            }
            frame "L" {
              n164 = call "DelayAutoLine.vi"() -> ()  [unwired: 12 in]
            }
          }
        }
      }
    }
    frame "Right Ln Ln Ln Ln" {
      n165 = flat-sequence {
        tunnel: w446 -> [w449]
        tunnel: [w449] -> w445
        tunnel: w445 -> [_]
        frame #0 {
          n166 = global write "Robot Global Data.vi" "Robot x Position"(277.0) -> ()
          n167 = global write "Robot Global Data.vi" "Robot y Position"(19.5) -> ()
        }
        frame #1 {
          n168 = call "DelayAutoLine.vi"() -> ()  [unwired: 12 in]
        }
      }
    }
    frame "Left Sw Sw Sw Sw" {
      n169 = flat-sequence {
        tunnel: w451 -> [w454]
        tunnel: [w454] -> w450
        tunnel: w450 -> [w455]
        frame #0 {
          n170 = global write "Robot Global Data.vi" "Robot y Position"(19.5) -> ()
          n171 = global write "Robot Global Data.vi" "Robot x Position"(46.0) -> ()
        }
        frame #1 {
          n172 = case shown="\"L\", Default" w455 {
            frame "R" {
              w456 = 0.3 ("power in")
              # "deliver to the far right side after going around back"
              n173 = call <vilib>:"WPI_RobotDriveRefNum Registry Get.vi"("refnum name"="Left and Right Motors") -> ("error out"=w480:errorcluster, "RobotDriveDevRef"=w481:T2)  [unwired: 9 in]
              n174 = call "Run by Point.vi"("end Power"=w456, "Power in"=w456, "error in (no error)"=w480, "y"=235.0, "x"=43.0, "RobotDriveDevRef"=w481) -> ("error out"=w472:errorcluster, "power out"=w471:dbl, "refnum"=w473:T2)  [unwired: 3 in]
              n175 = call "Turn to Angle.vi"("in power"=w471, "error in (no error)"=w472, "Angle"=90.0 ("x"), "RobotDriveDevRef"=w473) -> ("error out"=w467:errorcluster, "ref Num"=w466:T2)  [unwired: 5 in, 1 out]
              n176 = call "Run by Point.vi"("end Power"=w456, "Power in"=w456, "error in (no error)"=w467, "y"=235.0, "x"=281.0, "RobotDriveDevRef"=w466) -> ("error out"=w462:errorcluster, "power out"=w460:dbl, "refnum"=w463:T2)  [unwired: 3 in]
              n177 = call "Turn to Angle.vi"("in power"=w460, "error in (no error)"=w462, "Angle"=180.0, "RobotDriveDevRef"=w463) -> ("error out"=w470:errorcluster, "ref Num"=w469:T2)  [unwired: 5 in, 1 out]
              n178 = call "Run by Point.vi"("end Power"=0.0 ("final power"), "Power in"=w456, "error in (no error)"=w470, "y"=163.0, "x"=276.0, "RobotDriveDevRef"=w469) -> ("power out"=w458:dbl)  [unwired: 3 in, 2 out]
              n179 = call "Deliver Cube.vi"("run?"=w458, "Angle"=-90.0, "Scale?"=FALSE) -> ()  [unwired: 8 in, 1 out]
            }
            frame "L", Default {
              n180 = call <vilib>:"WPI_RobotDriveRefNum Registry Get.vi"("refnum name"="Left and Right Motors") -> ("error out"=w485:errorcluster, "RobotDriveDevRef"=w486:T2)  [unwired: 9 in]
              n181 = call "Run by Point.vi"("end Power"=0.0 ("final power"), "Power in"=0.0, "error in (no error)"=w485, "y"=163.0 ("x"), "x"=48.0 ("y"), "RobotDriveDevRef"=w486) -> ("power out"=w482:dbl)  [unwired: 3 in, 2 out]
              n182 = call "Deliver Cube.vi"("run?"=w482, "Angle"=90.0, "Scale?"=FALSE) -> ()  [unwired: 8 in, 1 out]
            }
          }
        }
      }
    }
    frame "Left Sc Sc Sc Sc" {
      n183 = flat-sequence {
        tunnel: [w493] -> w492
        tunnel: w492 -> [w499]
        frame #0 {
          n184 = global read "Robot Global Data.vi" "Game Data"() -> (w497:string)
          n185 = global write "Robot Global Data.vi" "Robot y Position"(19.5) -> ()
          n186 = global write "Robot Global Data.vi" "Robot x Position"(46.0) -> ()
          n187 = String Subset(string=w497, offset (0)=1, length (rest)=1 ("length (rest)")) -> (substring=w493:string)
        }
        frame #1 {
          n188 = case shown="\"R\"" w499 {
            frame "R" {
              w500 = 0.3 ("end Power")
              n189 = call <vilib>:"WPI_RobotDriveRefNum Registry Get.vi"("refnum name"="Left and Right Motors") -> ("error out"=w514:errorcluster, "RobotDriveDevRef"=w513:T2)  [unwired: 9 in]
              n190 = call "Run by Point.vi"("end Power"=w500, "Power in"=w500, "error in (no error)"=w514, "y"=235.0, "x"=43.0, "RobotDriveDevRef"=w513) -> ("error out"=w519:errorcluster, "power out"=w521:dbl, "refnum"=w515:T2)  [unwired: 3 in]
              n191 = call "Turn to Angle.vi"("in power"=w521, "error in (no error)"=w519, "Angle"=90.0, "RobotDriveDevRef"=w515) -> ("error out"=w520:errorcluster, "ref Num"=w516:T2)  [unwired: 5 in, 1 out]
              n192 = call "Run by Point.vi"("end Power"=w500, "Power in"=w500, "error in (no error)"=w520, "y"=235.0, "x"=281.0, "RobotDriveDevRef"=w516) -> ("error out"=w522:errorcluster, "power out"=w523:dbl, "refnum"=w518:T2)  [unwired: 3 in]
              n193 = call "Turn to Angle.vi"("in power"=w523, "error in (no error)"=w522, "Angle"=0.0, "RobotDriveDevRef"=w518) -> ("error out"=w524:errorcluster, "ref Num"=w517:T2)  [unwired: 5 in, 1 out]
              n194 = call "Run by Point.vi"("end Power"=w500, "Power in"=w500, "error in (no error)"=w524, "y"=300.0, "x"=288.0, "RobotDriveDevRef"=w517) -> ("power out"=w502:dbl)  [unwired: 3 in, 2 out]
              n195 = call "Deliver Cube.vi"("run?"=w502, "Angle"=-80.0, "Scale?"=TRUE) -> ()  [unwired: 8 in, 1 out]
            }
            frame "L", Default {
              w528 = 0.0 ("end Power")
              n196 = call <vilib>:"WPI_RobotDriveRefNum Registry Get.vi"("refnum name"="Left and Right Motors") -> ("error out"=w532:errorcluster, "RobotDriveDevRef"=w533:T2)  [unwired: 9 in]
              n197 = call "Run by Point.vi"("end Power"=w528, "Power in"=w528, "error in (no error)"=w532, "y"=263.0, "x"=87.0, "RobotDriveDevRef"=w533) -> ("power out"=w525:dbl)  [unwired: 3 in, 2 out]
              n198 = call "Deliver Cube.vi"("run?"=w525, "Angle"=5.0 ("in power"), "Scale?"=TRUE) -> ()  [unwired: 8 in, 1 out]
            }
          }
        }
      }
    }
    frame "Right Sc Sc Sc Sc" {
      n199 = flat-sequence {
        tunnel: [w535] -> w534
        tunnel: w534 -> [w541]
        frame #0 {
          n200 = global read "Robot Global Data.vi" "Game Data"() -> (w539:string)
          n201 = global write "Robot Global Data.vi" "Robot y Position"(19.5) -> ()
          n202 = global write "Robot Global Data.vi" "Robot x Position"(277.0) -> ()
          n203 = String Subset(string=w539, offset (0)=1, length (rest)=1 ("length (rest)")) -> (substring=w535:string)
        }
        frame #1 {
          n204 = case shown="\"L\"" w541 {
            frame "L" {
              w542 = 0.3 ("end Power")
              n205 = call <vilib>:"WPI_RobotDriveRefNum Registry Get.vi"("refnum name"="Left and Right Motors") -> ("error out"=w557:errorcluster, "RobotDriveDevRef"=w556:T2)  [unwired: 9 in]
              n206 = call "Run by Point.vi"("end Power"=w542, "Power in"=w542, "error in (no error)"=w557, "y"=235.0, "x"=281.0, "RobotDriveDevRef"=w556) -> ("error out"=w562:errorcluster, "power out"=w564:dbl, "refnum"=w558:T2)  [unwired: 3 in]
              n207 = call "Turn to Angle.vi"("in power"=w564, "error in (no error)"=w562, "Angle"=-90.0, "RobotDriveDevRef"=w558) -> ("error out"=w563:errorcluster, "out power"=w568:dbl, "ref Num"=w559:T2)  [unwired: 5 in]
              n208 = call "Run by Point.vi"("end Power"=w542, "Power in"=w568, "error in (no error)"=w563, "y"=235.0, "x"=43.0, "RobotDriveDevRef"=w559) -> ("error out"=w565:errorcluster, "power out"=w566:dbl, "refnum"=w561:T2)  [unwired: 3 in]
              n209 = call "Turn to Angle.vi"("in power"=w566, "error in (no error)"=w565, "Angle"=0.0, "RobotDriveDevRef"=w561) -> ("error out"=w567:errorcluster, "ref Num"=w560:T2)  [unwired: 5 in, 1 out]
              n210 = call "Run by Point.vi"("end Power"=0.0, "Power in"=w542, "error in (no error)"=w567, "y"=300.0, "x"=36.0, "RobotDriveDevRef"=w560) -> ("power out"=w544:dbl)  [unwired: 3 in, 2 out]
              n211 = call "Deliver Cube.vi"("run?"=w544, "Angle"=80.0, "Scale?"=TRUE) -> ()  [unwired: 8 in, 1 out]
            }
            frame "R", Default {
              w572 = 0.0 ("end Power")
              # "From Right Deliver to the near side of the Scale"
              n212 = call <vilib>:"WPI_RobotDriveRefNum Registry Get.vi"("refnum name"="Left and Right Motors") -> ("error out"=w576:errorcluster, "RobotDriveDevRef"=w577:T2)  [unwired: 9 in]
              n213 = call "Run by Point.vi"("end Power"=w572, "Power in"=w572, "error in (no error)"=w576, "y"=263.0, "x"=237.0, "RobotDriveDevRef"=w577) -> ("power out"=w569:dbl)  [unwired: 3 in, 2 out]
              n214 = call "Deliver Cube.vi"("run?"=w569, "Angle"=-5.0 ("in power"), "Scale?"=TRUE) -> ()  [unwired: 8 in, 1 out]
            }
          }
        }
      }
    }
    frame "Right Sw Sc Sw Sc" {
      n215 = flat-sequence {
        tunnel: [w582] -> w580
        tunnel: w579 -> [w582]
        tunnel: [w581] -> w578
        tunnel: w580 -> [_]
        tunnel: w578 -> [w587]
        frame #0 {
          n216 = global read "Robot Global Data.vi" "Game Data"() -> (w585:string)
          n217 = global write "Robot Global Data.vi" "Robot y Position"(19.5) -> ()
          n218 = global write "Robot Global Data.vi" "Robot x Position"(277.0) -> ()
          n219 = String Subset(string=w585, length (rest)=2 ("length (rest)")) -> (substring=w581:string)  [unwired: 1 in]
        }
        frame #1 {
          n220 = case shown="\"RR\"" w587 {
            frame "LL" {
              w588 = 0.3
              n221 = call <vilib>:"WPI_RobotDriveRefNum Registry Get.vi"("refnum name"="Left and Right Motors") -> ("error out"=w603:errorcluster, "RobotDriveDevRef"=w602:T2)  [unwired: 9 in]
              n222 = call "Run by Point.vi"("end Power"=w588, "Power in"=w588, "error in (no error)"=w603, "y"=235.0, "x"=281.0, "RobotDriveDevRef"=w602) -> ("error out"=w608:errorcluster, "power out"=w610:dbl, "refnum"=w604:T2)  [unwired: 3 in]
              n223 = call "Turn to Angle.vi"("in power"=w610, "error in (no error)"=w608, "Angle"=-90.0, "RobotDriveDevRef"=w604) -> ("error out"=w609:errorcluster, "out power"=w615:dbl, "ref Num"=w605:T2)  [unwired: 5 in]
              n224 = call "Run by Point.vi"("end Power"=w588, "Power in"=w615, "error in (no error)"=w609, "y"=235.0, "x"=43.0, "RobotDriveDevRef"=w605) -> ("error out"=w611:errorcluster, "power out"=w612:dbl, "refnum"=w607:T2)  [unwired: 3 in]
              n225 = call "Turn to Angle.vi"("in power"=w612, "error in (no error)"=w611, "Angle"=0.0, "RobotDriveDevRef"=w607) -> ("error out"=w613:errorcluster, "out power"=w614:dbl, "ref Num"=w606:T2)  [unwired: 5 in]
              n226 = call "Run by Point.vi"("end Power"=0.0, "Power in"=w614, "error in (no error)"=w613, "y"=300.0, "x"=36.0, "RobotDriveDevRef"=w606) -> ("power out"=w589:dbl)  [unwired: 3 in, 2 out]
              n227 = call "Deliver Cube.vi"("run?"=w589, "Angle"=80.0, "Scale?"=FALSE) -> ()  [unwired: 8 in, 1 out]
            }
            frame "RL" {
              w617 = 0.0 ("end Power")
              n228 = call <vilib>:"WPI_RobotDriveRefNum Registry Get.vi"("refnum name"="Left and Right Motors") -> ("error out"=w619:errorcluster, "RobotDriveDevRef"=w620:T2)  [unwired: 9 in]
              n229 = call "Run by Point.vi"("end Power"=w617, "Power in"=w617, "error in (no error)"=w619, "y"=163.0, "x"=276.0, "RobotDriveDevRef"=w620) -> ("power out"=w618:dbl)  [unwired: 3 in, 2 out]
              n230 = call "Deliver Cube.vi"("run?"=w618, "Angle"=-90.0 ("x"), "Scale?"=FALSE) -> ()  [unwired: 8 in, 1 out]
            }
            frame "LR", Default {
              w628 = 0.0 ("end Power")
              # "From Right Deliver to the near side of the Scale"
              n231 = call <vilib>:"WPI_RobotDriveRefNum Registry Get.vi"("refnum name"="Left and Right Motors") -> ("error out"=w632:errorcluster, "RobotDriveDevRef"=w633:T2)  [unwired: 9 in]
              n232 = call "Run by Point.vi"("end Power"=w628, "Power in"=w628, "error in (no error)"=w632, "y"=263.0, "x"=237.0, "RobotDriveDevRef"=w633) -> ("power out"=w625:dbl)  [unwired: 3 in, 2 out]
              n233 = call "Deliver Cube.vi"("run?"=w625, "Angle"=-5.0 ("in power"), "Scale?"=TRUE) -> ()  [unwired: 8 in, 1 out]
            }
            frame "RR" {
              w637 = 0.0 ("end Power")
              # "From Right Deliver to the near side of the Scale"
              n234 = call <vilib>:"WPI_RobotDriveRefNum Registry Get.vi"("refnum name"="Left and Right Motors") -> ("error out"=w641:errorcluster, "RobotDriveDevRef"=w642:T2)  [unwired: 9 in]
              n235 = call "Run by Point.vi"("end Power"=w637, "Power in"=w637, "error in (no error)"=w641, "y"=263.0, "x"=237.0, "RobotDriveDevRef"=w642) -> ("power out"=w634:dbl)  [unwired: 3 in, 2 out]
              n236 = call "Deliver Cube.vi"("run?"=w634, "Angle"=-5.0 ("in power"), "Scale?"=TRUE) -> ()  [unwired: 8 in, 1 out]
            }
          }
        }
      }
    }
    frame "Right Sw Sc Sw Sw" {
      n237 = flat-sequence {
        tunnel: [w647] -> w645
        tunnel: w644 -> [w647]
        tunnel: [w646] -> w643
        tunnel: w645 -> [_]
        tunnel: w643 -> [w652]
        frame #0 {
          n238 = global read "Robot Global Data.vi" "Game Data"() -> (w650:string)
          n239 = global write "Robot Global Data.vi" "Robot y Position"(19.5) -> ()
          n240 = global write "Robot Global Data.vi" "Robot x Position"(277.0) -> ()
          n241 = String Subset(string=w650, length (rest)=2 ("length (rest)")) -> (substring=w646:string)  [unwired: 1 in]
        }
        frame #1 {
          n242 = case shown="\"LR\", Default" w652 {
            frame "LL" {
              w653 = 0.3
              n243 = call <vilib>:"WPI_RobotDriveRefNum Registry Get.vi"("refnum name"="Left and Right Motors") -> ("error out"=w668:errorcluster, "RobotDriveDevRef"=w667:T2)  [unwired: 9 in]
              n244 = call "Run by Point.vi"("end Power"=w653, "Power in"=w653, "error in (no error)"=w668, "y"=235.0, "x"=281.0, "RobotDriveDevRef"=w667) -> ("error out"=w673:errorcluster, "power out"=w675:dbl, "refnum"=w669:T2)  [unwired: 3 in]
              n245 = call "Turn to Angle.vi"("in power"=w675, "error in (no error)"=w673, "Angle"=-90.0, "RobotDriveDevRef"=w669) -> ("error out"=w674:errorcluster, "ref Num"=w670:T2)  [unwired: 5 in, 1 out]
              n246 = call "Run by Point.vi"("end Power"=w653, "Power in"=w653, "error in (no error)"=w674, "y"=235.0, "x"=43.0, "RobotDriveDevRef"=w670) -> ("error out"=w676:errorcluster, "power out"=w677:dbl, "refnum"=w672:T2)  [unwired: 3 in]
              n247 = call "Turn to Angle.vi"("in power"=w677, "error in (no error)"=w676, "Angle"=0.0, "RobotDriveDevRef"=w672) -> ("error out"=w678:errorcluster, "ref Num"=w671:T2)  [unwired: 5 in, 1 out]
              n248 = call "Run by Point.vi"("end Power"=0.0, "Power in"=w653, "error in (no error)"=w678, "y"=300.0, "x"=36.0, "RobotDriveDevRef"=w671) -> ("power out"=w655:dbl)  [unwired: 3 in, 2 out]
              n249 = call "Deliver Cube.vi"("run?"=w655, "Angle"=80.0, "Scale?"=FALSE) -> ()  [unwired: 8 in, 1 out]
            }
            frame "RL" {
              w680 = 0.0 ("end Power")
              n250 = call <vilib>:"WPI_RobotDriveRefNum Registry Get.vi"("refnum name"="Left and Right Motors") -> ("error out"=w682:errorcluster, "RobotDriveDevRef"=w683:T2)  [unwired: 9 in]
              n251 = call "Run by Point.vi"("end Power"=w680, "Power in"=w680, "error in (no error)"=w682, "y"=163.0, "x"=276.0, "RobotDriveDevRef"=w683) -> ("power out"=w681:dbl)  [unwired: 3 in, 2 out]
              n252 = call "Deliver Cube.vi"("run?"=w681, "Angle"=-90.0 ("x"), "Scale?"=FALSE) -> ()  [unwired: 8 in, 1 out]
            }
            frame "LR", Default {
              w691 = 0.0 ("end Power")
              # "From Right Deliver to the near side of the Scale"
              n253 = call <vilib>:"WPI_RobotDriveRefNum Registry Get.vi"("refnum name"="Left and Right Motors") -> ("error out"=w695:errorcluster, "RobotDriveDevRef"=w696:T2)  [unwired: 9 in]
              n254 = call "Run by Point.vi"("end Power"=w691, "Power in"=w691, "error in (no error)"=w695, "y"=263.0, "x"=237.0, "RobotDriveDevRef"=w696) -> ("power out"=w688:dbl)  [unwired: 3 in, 2 out]
              n255 = call "Deliver Cube.vi"("run?"=w688, "Angle"=-5.0 ("in power"), "Scale?"=TRUE) -> ()  [unwired: 8 in, 1 out]
            }
            frame "RR" {
              w698 = 0.0 ("end Power")
              n256 = call <vilib>:"WPI_RobotDriveRefNum Registry Get.vi"("refnum name"="Left and Right Motors") -> ("error out"=w700:errorcluster, "RobotDriveDevRef"=w701:T2)  [unwired: 9 in]
              n257 = call "Run by Point.vi"("end Power"=w698, "Power in"=w698, "error in (no error)"=w700, "y"=163.0, "x"=276.0, "RobotDriveDevRef"=w701) -> ("power out"=w699:dbl)  [unwired: 3 in, 2 out]
              n258 = call "Deliver Cube.vi"("run?"=w699, "Angle"=-90.0 ("x"), "Scale?"=FALSE) -> ()  [unwired: 8 in, 1 out]
            }
          }
        }
      }
    }
    frame "Left Sc Sw Sc Sw" {
      n259 = flat-sequence {
        tunnel: [w710] -> w708
        tunnel: w707 -> [w710]
        tunnel: [w709] -> w706
        tunnel: w708 -> [_]
        tunnel: w706 -> [w715]
        frame #0 {
          n260 = global read "Robot Global Data.vi" "Game Data"() -> (w713:string)
          n261 = global write "Robot Global Data.vi" "Robot y Position"(19.5) -> ()
          n262 = global write "Robot Global Data.vi" "Robot x Position"(46.0) -> ()
          n263 = String Subset(string=w713, length (rest)=2 ("length (rest)")) -> (substring=w709:string)  [unwired: 1 in]
        }
        frame #1 {
          n264 = case shown="\"LL\"" w715 {
            frame "LL" {
              w719 = 0.0 ("end Power")
              # "From Left Deliver to the near side of the Scale"
              n265 = call <vilib>:"WPI_RobotDriveRefNum Registry Get.vi"("refnum name"="Left and Right Motors") -> ("error out"=w723:errorcluster, "RobotDriveDevRef"=w724:T2)  [unwired: 9 in]
              n266 = call "Run by Point.vi"("end Power"=w719, "Power in"=w719, "error in (no error)"=w723, "y"=263.0, "x"=87.0, "RobotDriveDevRef"=w724) -> ("power out"=w716:dbl)  [unwired: 3 in, 2 out]
              n267 = call "Deliver Cube.vi"("run?"=w716, "Angle"=5.0 ("in power"), "Scale?"=TRUE) -> ()  [unwired: 8 in, 1 out]
            }
            frame "RL" {
              w728 = 0.0 ("end Power")
              n268 = call <vilib>:"WPI_RobotDriveRefNum Registry Get.vi"("refnum name"="Left and Right Motors") -> ("error out"=w732:errorcluster, "RobotDriveDevRef"=w733:T2)  [unwired: 9 in]
              n269 = call "Run by Point.vi"("end Power"=w728, "Power in"=w728, "error in (no error)"=w732, "y"=300.0, "x"=36.0, "RobotDriveDevRef"=w733) -> ("power out"=w725:dbl)  [unwired: 3 in, 2 out]
              n270 = call "Deliver Cube.vi"("run?"=w725, "Angle"=80.0 ("in power"), "Scale?"=TRUE) -> ()  [unwired: 8 in, 1 out]
            }
            frame "LR", Default {
              w737 = 0.0 ("end Power")
              # "From Left Deliver to the near side of the Scale"
              n271 = call <vilib>:"WPI_RobotDriveRefNum Registry Get.vi"("refnum name"="Left and Right Motors") -> ("error out"=w741:errorcluster, "RobotDriveDevRef"=w742:T2)  [unwired: 9 in]
              n272 = call "Run by Point.vi"("end Power"=w737, "Power in"=w737, "error in (no error)"=w741, "y"=263.0, "x"=87.0, "RobotDriveDevRef"=w742) -> ("power out"=w734:dbl)  [unwired: 3 in, 2 out]
              n273 = call "Deliver Cube.vi"("run?"=w734, "Angle"=5.0 ("in power"), "Scale?"=TRUE) -> ()  [unwired: 8 in, 1 out]
            }
            frame "RR" {
              w743 = 0.3 ("end Power")
              # "deliver to the far right switch after going around back"
              n274 = call <vilib>:"WPI_RobotDriveRefNum Registry Get.vi"("refnum name"="Left and Right Motors") -> ("error out"=w767:errorcluster, "RobotDriveDevRef"=w768:T2)  [unwired: 9 in]
              n275 = call "Run by Point.vi"("end Power"=w743, "Power in"=w743, "error in (no error)"=w767, "y"=235.0, "x"=43.0, "RobotDriveDevRef"=w768) -> ("error out"=w758:errorcluster, "power out"=w757:dbl, "refnum"=w759:T2)  [unwired: 3 in]
              n276 = call "Turn to Angle.vi"("in power"=w757, "error in (no error)"=w758, "Angle"=90.0 ("x"), "RobotDriveDevRef"=w759) -> ("error out"=w753:errorcluster, "ref Num"=w752:T2)  [unwired: 5 in, 1 out]
              n277 = call "Run by Point.vi"("end Power"=w743, "Power in"=w743, "error in (no error)"=w753, "y"=235.0, "x"=281.0, "RobotDriveDevRef"=w752) -> ("error out"=w748:errorcluster, "power out"=w746:dbl, "refnum"=w749:T2)  [unwired: 3 in]
              n278 = call "Turn to Angle.vi"("in power"=w746, "error in (no error)"=w748, "Angle"=180.0, "RobotDriveDevRef"=w749) -> ("error out"=w756:errorcluster, "ref Num"=w755:T2)  [unwired: 5 in, 1 out]
              n279 = call "Run by Point.vi"("end Power"=0.0 ("final power"), "Power in"=w743, "error in (no error)"=w756, "y"=163.0, "x"=276.0, "RobotDriveDevRef"=w755) -> ("power out"=w744:dbl)  [unwired: 3 in, 2 out]
              n280 = call "Deliver Cube.vi"("run?"=w744, "Angle"=-90.0, "Scale?"=FALSE) -> ()  [unwired: 8 in, 1 out]
            }
          }
        }
      }
    }
    frame "Left Sw Sw Sc Sw" {
      n281 = flat-sequence {
        tunnel: [w773] -> w771
        tunnel: w770 -> [w773]
        tunnel: [w772] -> w769
        tunnel: w771 -> [_]
        tunnel: w769 -> [w778]
        frame #0 {
          n282 = global read "Robot Global Data.vi" "Game Data"() -> (w776:string)
          n283 = global write "Robot Global Data.vi" "Robot y Position"(19.5) -> ()
          n284 = global write "Robot Global Data.vi" "Robot x Position"(46.0) -> ()
          n285 = String Subset(string=w776, length (rest)=2 ("length (rest)")) -> (substring=w772:string)  [unwired: 1 in]
        }
        frame #1 {
          n286 = case shown="\"RL\"" w778 {
            frame "LL" {
              n287 = call <vilib>:"WPI_RobotDriveRefNum Registry Get.vi"("refnum name"="Left and Right Motors") -> ("error out"=w782:errorcluster, "RobotDriveDevRef"=w783:T2)  [unwired: 9 in]
              n288 = call "Run by Point.vi"("end Power"=0.0 ("final power"), "Power in"=0.0, "error in (no error)"=w782, "y"=163.0 ("x"), "x"=48.0 ("y"), "RobotDriveDevRef"=w783) -> ("power out"=w779:dbl)  [unwired: 3 in, 2 out]
              n289 = call "Deliver Cube.vi"("run?"=w779, "Angle"=90.0, "Scale?"=FALSE) -> ()  [unwired: 8 in, 1 out]
            }
            frame "RL" {
              w792 = 0.0 ("end Power")
              # "From Left Deliver to the near side of the Scale"
              n290 = call <vilib>:"WPI_RobotDriveRefNum Registry Get.vi"("refnum name"="Left and Right Motors") -> ("error out"=w796:errorcluster, "RobotDriveDevRef"=w797:T2)  [unwired: 9 in]
              n291 = call "Run by Point.vi"("end Power"=w792, "Power in"=w792, "error in (no error)"=w796, "y"=263.0, "x"=87.0, "RobotDriveDevRef"=w797) -> ("power out"=w789:dbl)  [unwired: 3 in, 2 out]
              n292 = call "Deliver Cube.vi"("run?"=w789, "Angle"=5.0 ("in power"), "Scale?"=TRUE) -> ()  [unwired: 8 in, 1 out]
            }
            frame "LR", Default {
              n293 = call <vilib>:"WPI_RobotDriveRefNum Registry Get.vi"("refnum name"="Left and Right Motors") -> ("error out"=w801:errorcluster, "RobotDriveDevRef"=w802:T2)  [unwired: 9 in]
              n294 = call "Run by Point.vi"("end Power"=0.0 ("final power"), "Power in"=0.0, "error in (no error)"=w801, "y"=163.0 ("x"), "x"=48.0 ("y"), "RobotDriveDevRef"=w802) -> ("power out"=w798:dbl)  [unwired: 3 in, 2 out]
              n295 = call "Deliver Cube.vi"("run?"=w798, "Angle"=90.0, "Scale?"=FALSE) -> ()  [unwired: 8 in, 1 out]
            }
            frame "RR" {
              w808 = 0.3 ("end Power")
              # "deliver to the far right side after going around back"
              n296 = call <vilib>:"WPI_RobotDriveRefNum Registry Get.vi"("refnum name"="Left and Right Motors") -> ("error out"=w831:errorcluster, "RobotDriveDevRef"=w832:T2)  [unwired: 9 in]
              n297 = call "Run by Point.vi"("end Power"=w808, "Power in"=w808, "error in (no error)"=w831, "y"=235.0, "x"=43.0, "RobotDriveDevRef"=w832) -> ("error out"=w823:errorcluster, "power out"=w822:dbl, "refnum"=w824:T2)  [unwired: 3 in]
              n298 = call "Turn to Angle.vi"("in power"=w822, "error in (no error)"=w823, "Angle"=90.0 ("x"), "RobotDriveDevRef"=w824) -> ("error out"=w818:errorcluster, "ref Num"=w817:T2)  [unwired: 5 in, 1 out]
              n299 = call "Run by Point.vi"("end Power"=w808, "Power in"=w808, "error in (no error)"=w818, "y"=235.0, "x"=281.0, "RobotDriveDevRef"=w817) -> ("error out"=w813:errorcluster, "power out"=w811:dbl, "refnum"=w814:T2)  [unwired: 3 in]
              n300 = call "Turn to Angle.vi"("in power"=w811, "error in (no error)"=w813, "Angle"=180.0, "RobotDriveDevRef"=w814) -> ("error out"=w821:errorcluster, "ref Num"=w820:T2)  [unwired: 5 in, 1 out]
              n301 = call "Run by Point.vi"("end Power"=w808, "Power in"=w808, "error in (no error)"=w821, "y"=163.0, "x"=276.0, "RobotDriveDevRef"=w820) -> ("power out"=w809:dbl)  [unwired: 3 in, 2 out]
              n302 = call "Deliver Cube.vi"("run?"=w809, "Angle"=-90.0, "Scale?"=FALSE) -> ()  [unwired: 8 in, 1 out]
            }
          }
        }
      }
    }
    frame "Center Two Cube" {
      n303 = flat-sequence {
        tunnel: w833 -> [w837]
        tunnel: [w837] -> w834
        tunnel: w834 -> [w838]
        frame #0 {
          n304 = global write "Robot Global Data.vi" "Robot y Position"(19.5) -> ()
          n305 = global write "Robot Global Data.vi" "Robot x Position"(167.0) -> ()
        }
        frame #1 {
          n306 = case shown="\"R\"" w838 {
            frame "R" {
              w839 = 0.3 ("end Power")
              w840 = 0.3 ("end Power")
              n307 = call <vilib>:"WPI_RobotDriveRefNum Registry Get.vi"("refnum name"="Left and Right Motors") -> ("error out"=w867:errorcluster, "RobotDriveDevRef"=w868:T2)  [unwired: 9 in]
              n308 = call "Run by Point.vi"("end Power"=0.0, "Power in"=0.2, "error in (no error)"=w867, "y"=103.0, "x"=216.0, "RobotDriveDevRef"=w868) -> ("error out"=w842:errorcluster, "power out"=w866:dbl, "refnum"=w843:T2)  [unwired: 3 in]
              n309 = call "Deliver Cube.vi"("run?"=w866, "Angle"=0.0, "Scale?"=FALSE) -> ()  [unwired: 8 in, 1 out]
              n310 = call "Run by Point.vi"("end Power"=w840, "Power in"=w840, "error in (no error)"=w842, "y"=53.0, "x"=162.0, "RobotDriveDevRef"=w843) -> ("error out"=w858:errorcluster, "power out"=w841:dbl, "refnum"=w859:T2)  [unwired: 3 in]
              n311 = while {
                tunnel: w841 -> [_]
                stop <- TRUE stop-if-true
                n312 = global write "Robot Global Data.vi" "Intake?"("In" ("Intake?")) -> ()
                n313 = global write "Robot Global Data.vi" "Open?"(TRUE ("Open?")) -> ()
              }
              n314 = call "Turn to Angle.vi"("in power"=w841, "error in (no error)"=w858, "Angle"=0.0, "RobotDriveDevRef"=w859) -> ("error out"=w857:errorcluster, "ref Num"=w856:T2)  [unwired: 5 in, 1 out]
              n315 = call "Run by Point.vi"("end Power"=w839, "Power in"=w839, "error in (no error)"=w857, "y"=81.5, "x"=162.0, "RobotDriveDevRef"=w856) -> ("error out"=w851:errorcluster, "power out"=w850:dbl, "refnum"=w852:T2)  [unwired: 3 in]
              n316 = while {
                tunnel: w850 -> [w872]
                stop <- TRUE stop-if-true
                n317 = flat-sequence {
                  tunnel: w872 -> [_]
                  frame #0 {
                    n318 = global write "Robot Global Data.vi" "Open?"(FALSE ("Open?")) -> ()
                    n319 = Wait (ms)(milliseconds to wait=u32 300) -> ()  [unwired: 1 out]
                  }
                  frame #1 {
                    n320 = global write "Robot Global Data.vi" "Intake?"("Neutral" ("Intake?")) -> ()
                  }
                }
              }
              n321 = call "Run by Point.vi"("end Power"=0.0, "Power in"=w839, "error in (no error)"=w851, "y"=103.0, "x"=216.0, "RobotDriveDevRef"=w852) -> ("power out"=w846:dbl)  [unwired: 3 in, 2 out]
              n322 = call "Deliver Cube.vi"("run?"=w846, "Angle"=0.0, "Scale?"=FALSE) -> ()  [unwired: 8 in, 1 out]
            }
            frame "L", Default {
              w880 = 0.3 ("end Power")
              n323 = call <vilib>:"WPI_RobotDriveRefNum Registry Get.vi"("refnum name"="Left and Right Motors") -> ("error out"=w909:errorcluster, "RobotDriveDevRef"=w910:T2)  [unwired: 9 in]
              n324 = call "Run by Point.vi"("end Power"=0.0, "Power in"=0.35, "error in (no error)"=w909, "y"=103.0, "x"=108.0, "RobotDriveDevRef"=w910) -> ("error out"=w902:errorcluster, "power out"=w904:dbl, "refnum"=w903:T2)  [unwired: 3 in]
              n325 = call "Deliver Cube.vi"("run?"=w904, "Angle"=0.0, "Scale?"=FALSE) -> ("out"=w898:dbl)  [unwired: 8 in]
              n326 = call "Run by Point.vi"("end Power"=0.3, "Power in"=w898, "error in (no error)"=w902, "y"=55.0, "x"=162.0, "RobotDriveDevRef"=w903) -> ("error out"=w896:errorcluster, "power out"=w881:dbl, "refnum"=w897:T2)  [unwired: 3 in]
              n327 = while {
                tunnel: [w920] -> _
                tunnel: w881 -> [w920]
                stop <- TRUE stop-if-true
                n328 = global write "Robot Global Data.vi" "Open?"(TRUE ("Open?")) -> ()
                n329 = global write "Robot Global Data.vi" "Intake?"("In" ("Intake?")) -> ()
              }
              n330 = call "Turn to Angle.vi"("in power"=w881, "error in (no error)"=w896, "Angle"=0.0, "RobotDriveDevRef"=w897) -> ("error out"=w895:errorcluster, "ref Num"=w894:T2)  [unwired: 5 in, 1 out]
              n331 = call "Run by Point.vi"("end Power"=w880, "Power in"=w880, "error in (no error)"=w895, "y"=81.5, "x"=162.0, "RobotDriveDevRef"=w894) -> ("error out"=w889:errorcluster, "power out"=w888:dbl, "refnum"=w890:T2)  [unwired: 3 in]
              n332 = while {
                tunnel: w888 -> [w914]
                stop <- TRUE stop-if-true
                n333 = flat-sequence {
                  tunnel: w914 -> [_]
                  frame #0 {
                    n334 = global write "Robot Global Data.vi" "Open?"(FALSE ("Open?")) -> ()
                    n335 = Wait (ms)(milliseconds to wait=u32 300) -> ()  [unwired: 1 out]
                  }
                  frame #1 {
                    n336 = global write "Robot Global Data.vi" "Intake?"("Neutral" ("Intake?")) -> ()
                  }
                }
              }
              n337 = call "Run by Point.vi"("end Power"=0.0, "Power in"=w888, "error in (no error)"=w889, "y"=103.0, "x"=108.0, "RobotDriveDevRef"=w890) -> ("power out"=w884:dbl)  [unwired: 3 in, 2 out]
              n338 = call "Deliver Cube.vi"("run?"=w884, "Angle"=0.0, "Scale?"=FALSE) -> ()  [unwired: 8 in, 1 out]
            }
          }
        }
      }
    }
  }
  n339 = while {
    stop <- w923 stop-if-true
    n340 = global read "Robot Global Data.vi" "Hoist Position"() -> (w925:string)
    n341 = case shown="\"Switch\"" w925 {
      frame "Scale" {
        n342 = call <vilib>:"CTRE_Phoenix_MotorControl_RefNumRegistryGet.vi"("refnum name"="Master Hoist") -> ("error out"=w939:errorcluster, "PhoenixMotorControlDevRef"=w938:T3)  [unwired: 9 in]
        n343 = call-poly <vilib>:"CTRE_Phoenix_MotorController_Get_Enhanced.vi"("PhoenixMotorControlDevRef"=w938, "error in"=w939) -> ("Quadrature Position"=w926:i32)  [unwired: 10 in, 3 out]
        n344 = Divide(x=w926, y=395.0) -> (x/y=w934:dbl)
        n345 = Subtract(x=w934, y=70.0) -> (x-y=w929:dbl)
        n346 = call "scale to range.vi"("Max"=0.8, "High"=-6.0, "Min"=-0.2, "Low"=6.0, "In Signal"=w929) -> ("Output signal"=w927:dbl)  [unwired: 6 in]
        n347 = call <vilib>:"WPI_RobotDriveRefNum Registry Get.vi"("refnum name"="Hoist") -> ("error out"=w941:errorcluster, "RobotDriveDevRef"=w935:T2)  [unwired: 9 in]
        n348 = call <vilib>:"WPI_RobotDriveTankDrive.vi"("error in (no error)"=w941, "Right axis value"=w927, "Left axis value"=w927, "RobotDriveDevRef"=w935) -> ()  [unwired: 5 in, 3 out]
      }
      frame "Pickup", Default {
        n349 = call <vilib>:"CTRE_Phoenix_MotorControl_RefNumRegistryGet.vi"("refnum name"="Master Hoist") -> ("error out"=w953:errorcluster, "PhoenixMotorControlDevRef"=w952:T3)  [unwired: 9 in]
        n350 = call-poly <vilib>:"CTRE_Phoenix_MotorController_Get_Enhanced.vi"("PhoenixMotorControlDevRef"=w952, "error in"=w953) -> ("Quadrature Position"=w942:i32)  [unwired: 10 in, 3 out]
        n351 = Divide(x=w942, y=395.0) -> (x/y=w944:dbl)
        n352 = call "scale to range.vi"("Max"=0.1, "High"=1.0, "Min"=-0.25, "Low"=3.0, "In Signal"=w944) -> ("Output signal"=w943:dbl)  [unwired: 6 in]
        n353 = call <vilib>:"WPI_RobotDriveRefNum Registry Get.vi"("refnum name"="Hoist") -> ("error out"=w955:errorcluster, "RobotDriveDevRef"=w949:T2)  [unwired: 9 in]
        n354 = call <vilib>:"WPI_RobotDriveTankDrive.vi"("error in (no error)"=w955, "Right axis value"=w943, "Left axis value"=w943, "RobotDriveDevRef"=w949) -> ()  [unwired: 5 in, 3 out]
      }
      frame "Switch" {
        n355 = call <vilib>:"CTRE_Phoenix_MotorControl_RefNumRegistryGet.vi"("refnum name"="Master Hoist") -> ("error out"=w969:errorcluster, "PhoenixMotorControlDevRef"=w968:T3)  [unwired: 9 in]
        n356 = call-poly <vilib>:"CTRE_Phoenix_MotorController_Get_Enhanced.vi"("PhoenixMotorControlDevRef"=w968, "error in"=w969) -> ("Quadrature Position"=w956:i32)  [unwired: 10 in, 3 out]
        n357 = Divide(x=w956, y=395.0) -> (x/y=w964:dbl)
        n358 = Subtract(x=w964, y=25.0) -> (x-y=w957:dbl)
        n359 = call "scale to range.vi"("Max"=0.8, "High"=-4.0, "Min"=-0.25, "Low"=4.0, "In Signal"=w957) -> ("Output signal"=w958:dbl)  [unwired: 6 in]
        n360 = call <vilib>:"WPI_RobotDriveRefNum Registry Get.vi"("refnum name"="Hoist") -> ("error out"=w971:errorcluster, "RobotDriveDevRef"=w965:T2)  [unwired: 9 in]
        n361 = call <vilib>:"WPI_RobotDriveTankDrive.vi"("error in (no error)"=w971, "Right axis value"=w958, "Left axis value"=w958, "RobotDriveDevRef"=w965) -> ()  [unwired: 5 in, 3 out]
      }
    }
    n362 = Wait (ms)(milliseconds to wait=u32 20) -> ()  [unwired: 1 out]
    n363 = call "stop.vi"() -> ("Boolean"=w923:bool)  [unwired: 11 in]
  }
  n364 = while {
    stop <- w973 stop-if-true
    n365 = Tick Count (ms)() -> (millisecond timer value=w974:u32)
    n366 = Wait (ms)(milliseconds to wait=u32 20) -> ()  [unwired: 1 out]
    n367 = while {
      tunnel: w974 -> [w982]
      stop <- w975 stop-if-true
      n368 = Tick Count (ms)() -> (millisecond timer value=w981:u32)
      n369 = global read "Robot Global Data.vi" "Tilt Time"() -> (w979:dbl)
      n370 = Wait (ms)(milliseconds to wait=u32 10) -> ()  [unwired: 1 out]
      n371 = Subtract(x=w981, y=w982) -> (x-y=w980:u32)
      n372 = Greater Or Equal?(x=w980, y=w979) -> (x >= y?=w978:bool)
      n373 = call "stop.vi"() -> ("Boolean"=w977:bool)  [unwired: 11 in]
      n374 = Or(x=w978, y=w977) -> (x .or. y?=w976:bool)
      n375 = case shown="False" w976 {
        selector: w976 -> [w984 w999]
        tunnel: [w984 w999] -> w975
        frame False {
          n376 = global read "Robot Global Data.vi" "Tilt Control"() -> (w985:string)
          n377 = case shown="\"Neutral\", Default" w985 {
            frame "Down" {
              n378 = call <vilib>:"WPI_MotorControlRefNum Registry Get.vi"("refnum name"="Tilt") -> ("error out"=w986:errorcluster, "MotorControlDevRef"=w989:T3)  [unwired: 9 in]
              n379 = call <vilib>:"WPI_MotorControlSetOutput.vi"("error in (no error)"=w986, "Output"=-0.6, "MotorControlDevRef"=w989) -> ()  [unwired: 6 in, 3 out]
            }
            frame "Neutral", Default {
              n380 = call <vilib>:"WPI_MotorControlRefNum Registry Get.vi"("refnum name"="Tilt") -> ("error out"=w993:errorcluster, "MotorControlDevRef"=w992:T3)  [unwired: 9 in]
              n381 = call <vilib>:"WPI_MotorControlSetOutput.vi"("error in (no error)"=w993, "Output"=0.0, "MotorControlDevRef"=w992) -> ()  [unwired: 6 in, 3 out]
            }
            frame "Up" {
              n382 = call <vilib>:"WPI_MotorControlRefNum Registry Get.vi"("refnum name"="Tilt") -> ("error out"=w994:errorcluster, "MotorControlDevRef"=w997:T3)  [unwired: 9 in]
              n383 = call <vilib>:"WPI_MotorControlSetOutput.vi"("error in (no error)"=w994, "Output"=1.0, "MotorControlDevRef"=w997) -> ()  [unwired: 6 in, 3 out]
            }
          }
        }
        frame True {
          n384 = global write "Robot Global Data.vi" "Tilt Time"(0.0 ("Tilt Time")) -> ()
          n385 = global write "Robot Global Data.vi" "Tilt Control"("Neutral" ("Tilt Control")) -> ()
          n386 = call <vilib>:"WPI_MotorControlRefNum Registry Get.vi"("refnum name"="Tilt") -> ("error out"=w998:errorcluster, "MotorControlDevRef"=w1003:T3)  [unwired: 9 in]
          n387 = call <vilib>:"WPI_MotorControlSetOutput.vi"("error in (no error)"=w998, "Output"=0.0, "MotorControlDevRef"=w1003) -> ()  [unwired: 6 in, 3 out]
        }
      }
    }
    n388 = call "stop.vi"() -> ("Boolean"=w973:bool)  [unwired: 11 in]
  }
  n389 = while {
    stop <- w1006 stop-if-true
    n390 = global read "Robot Global Data.vi" "Intake?"() -> (w1007:string)
    n391 = global read "Robot Global Data.vi" "Open?"() -> (w1011:bool)
    n392 = Wait (ms)(milliseconds to wait=u32 20) -> ()  [unwired: 1 out]
    n393 = Select(t=WPI_SolenoidValue."On" ("Value"), s=w1011, f=WPI_SolenoidValue."Off" ("Value")) -> (s? t:f=w1008:T1)
    n394 = case shown="\"In\"" w1007 {
      frame "In" {
        w1015 = 0.5
        n395 = call <vilib>:"WPI_MotorControlRefNum Registry Get.vi"("refnum name"="Left intake") -> ("error out"=w1019:errorcluster, "MotorControlDevRef"=w1018:T3)  [unwired: 9 in]
        n396 = call <vilib>:"WPI_MotorControlRefNum Registry Get.vi"("refnum name"="Right intake") -> ("error out"=w1021:errorcluster, "MotorControlDevRef"=w1020:T3)  [unwired: 9 in]
        n397 = call <vilib>:"WPI_MotorControlSetOutput.vi"("error in (no error)"=w1019, "Output"=w1015, "MotorControlDevRef"=w1018) -> ()  [unwired: 6 in, 3 out]
        n398 = call <vilib>:"WPI_MotorControlSetOutput.vi"("error in (no error)"=w1021, "Output"=w1015, "MotorControlDevRef"=w1020) -> ()  [unwired: 6 in, 3 out]
      }
      frame "Neutral", Default {
        w1022 = 0.0
        n399 = call <vilib>:"WPI_MotorControlRefNum Registry Get.vi"("refnum name"="Left intake") -> ("error out"=w1026:errorcluster, "MotorControlDevRef"=w1025:T3)  [unwired: 9 in]
        n400 = call <vilib>:"WPI_MotorControlRefNum Registry Get.vi"("refnum name"="Right intake") -> ("error out"=w1028:errorcluster, "MotorControlDevRef"=w1027:T3)  [unwired: 9 in]
        n401 = call <vilib>:"WPI_MotorControlSetOutput.vi"("error in (no error)"=w1026, "Output"=w1022, "MotorControlDevRef"=w1025) -> ()  [unwired: 6 in, 3 out]
        n402 = call <vilib>:"WPI_MotorControlSetOutput.vi"("error in (no error)"=w1028, "Output"=w1022, "MotorControlDevRef"=w1027) -> ()  [unwired: 6 in, 3 out]
      }
      frame "Out" {
        w1029 = -0.6
        n403 = call <vilib>:"WPI_MotorControlRefNum Registry Get.vi"("refnum name"="Left intake") -> ("error out"=w1033:errorcluster, "MotorControlDevRef"=w1032:T3)  [unwired: 9 in]
        n404 = call <vilib>:"WPI_MotorControlRefNum Registry Get.vi"("refnum name"="Right intake") -> ("error out"=w1035:errorcluster, "MotorControlDevRef"=w1034:T3)  [unwired: 9 in]
        n405 = call <vilib>:"WPI_MotorControlSetOutput.vi"("error in (no error)"=w1033, "Output"=w1029, "MotorControlDevRef"=w1032) -> ()  [unwired: 6 in, 3 out]
        n406 = call <vilib>:"WPI_MotorControlSetOutput.vi"("error in (no error)"=w1035, "Output"=w1029, "MotorControlDevRef"=w1034) -> ()  [unwired: 6 in, 3 out]
      }
    }
    n407 = call <vilib>:"WPI_SolenoidRefNum Registry Get.vi"("refnum name"="tele clamp") -> ("error out"=w1014:errorcluster, "SolenoidDevRef"=w1012:T9)  [unwired: 9 in]
    n408 = call-poly <vilib>:"WPI_SolenoidSet.vi"("error in (no error)"=w1014, "Value"=w1008, "SolenoidDevRef"=w1012) -> ()  [unwired: 7 in, 2 out]
    n409 = call "stop.vi"() -> ("Boolean"=w1006:bool)  [unwired: 11 in]
  }
